vi "CreatePaths_OpenFiles.vi"(8 "error in (no error)":errorcluster, 11 "HDF5_file_refs in":T2={"base path"=path "", "PathNow1"=path "", "PathNow2"=path "", "DateNow"="", "NAS path"=path "", "LogFiltStage"=FALSE, "LogNoise_df_1"=FALSE, "LogNoise_df_2"=FALSE, "LogNoise_df_3"=FALSE, "LogNoise_df_4"=FALSE, "Config"={"UsrCfg"={"Paths"={"CfgFile"=path "", "LogFolder"=path "", "LogFile"=path "", "NAS path"=path "", "ThreshFile"=path "", "RedunFolder"=path ""}, "SampleRate"=0.0}, "FP_User"={"#NoiseSums"=0, "Max_df"=1, "AvgAvg"=FALSE, "#Avg"=0, "AutoCenter"=FALSE, "Inclin"={"Vmin"=0.0, "Vmax"=0.0, "Angle_min"=0.0, "Angle_max"=0.0, "Offset"=0.0, "Pos_Neg"=FALSE}, "1"={"Cal_"={"Fine"=0.0, "Coarse_"=0.0}, "Beac"={"Fine"=0.0, "Coarse_"=0.0}, "Scale"={"Step4"=0.0, "Step5"=0.0, "Step6"=0.0, "Step7"=0.0}, "Offset"=0.0, "Scale_Noise"=0.0, "Scale_Step1"=0.0, "Scale_In_RT"=0.0, "ScaleMeas"=0.0, "FreqsToRemove"=[], "Width"=[0, 1633], "ScaleMeasEnum"=enum."1", "FilterEnab"=enum."Step 1"}, "2"={"Cal_"={"Fine"=0.0, "Coarse_"=0.0}, "Beac"={"Fine"=0.0, "Coarse_"=0.0}, "Scale"={"Step4"=0.0, "Step5"=0.0, "Step6"=0.0, "Step7"=0.0}, "Offset"=0.0, "Scale_Noise"=0.0, "Scale_Step1"=0.0, "Scale_In_RT"=0.0, "ScaleMeas"=0.0, "FreqsToRemove"=[], "Width"=[0, 1633], "ScaleMeasEnum"=enum."1", "FilterEnab"=enum."Step 1"}, "3"={"Cal_"={"Fine"=0.0, "Coarse_"=0.0}, "Beac"={"Fine"=0.0, "Coarse_"=0.0}, "Scale"={"Step4"=0.0, "Step5"=0.0, "Step6"=0.0, "Step7"=0.0}, "Offset"=0.0, "Scale_Noise"=0.0, "Scale_Step1"=0.0, "Scale_In_RT"=0.0, "ScaleMeas"=0.0, "FreqsToRemove"=[], "Width"=[0, 1633], "ScaleMeasEnum"=enum."1", "FilterEnab"=enum."Step 1"}, "4"={"Cal_"={"Fine"=0.0, "Coarse_"=0.0}, "Beac"={"Fine"=0.0, "Coarse_"=0.0}, "Scale"={"Step4"=0.0, "Step5"=0.0, "Step6"=0.0, "Step7"=0.0}, "Offset"=0.0, "Scale_Noise"=0.0, "Scale_Step1"=0.0, "Scale_In_RT"=0.0, "ScaleMeas"=0.0, "FreqsToRemove"=[], "Width"=[0, 1633], "ScaleMeasEnum"=enum."1", "FilterEnab"=enum."Step 1"}, "Target to Probe"=enum."1", "SNR_Thresh"=0.0, "Paths"={"CfgFile"=path "", "LogFolder"=path "", "LogFile"=path "", "NAS path"=path "", "ThreshFile"=path "", "RedunFolder"=path ""}, "Connex_Location"="", "SimulateFPGA"=FALSE, "Deadband"=0.0}}, "HDFRefs1"={"File"=0, "ToneRefs"=[], "NoiseRefs"=[], "TC_Refs"={"Group_ref"=0, "TimeString_dset"=0, "TimeStamp_dset"=0, "TC0_LP1_Hi"=0, "TC1_LP1_MidHi"=0, "TC2_LP1_Mid"=0, "TC3_LP1_LoMid"=0, "TC4_LP1_Lo"=0, "TC5_LP2_Hi"=0, "TC6_LP2_MidHi"=0, "TC7_LP2_Mid"=0, "TC8_LP2_LoMid"=0, "TC9_LP2_Lo"=0, "TC10_HVAC_Cond_In"=0, "TC11_HVAC_Cond_Out"=0, "TC12_Gen_Exhaust"=0, "TC13_Tamb_Inter"=0}, "ValidRefs"={"Group_ref"=0, "Weath_Valid_dset"=0, "Disdr_Valid_dset"=0, "Saturat_dset"=0, "Alarm_Valid_dset"=0, "Time_Valid_dset"=0, "Time_AlarmChange_dset"=0, "Alarm_Source_dset"=0}, "DisdromRefs"={"BasicGroup_ref"=0, "TimeStamp_dset"=0, "TotalRainRate_dset"=0, "Liquid_dset"=0, "Solid_dset"=0, "TotalRain_dset"=0, "Visibility_dset"=0, "RadarReflect_dset"=0, "MaxDiam_dset"=0, "MeasdParticles_dset"=0, "ParticlMinSpeed_dset"=0, "ParticlMaxSpeed_dset"=0, "ParticlMinDiam_dset"=0, "NonHydrParticls_dset"=0, "NonHydrVolum_dset"=0, "UnknownParticls_dset"=0, "UnknownVolum_dset"=0, "HydromType_dset"=0, "SpectGroup_ref"=0, "Spectrum_dset"=0, "Status_dset_deprecated"=0}, "TE_Refs"={"Group_ref"=0, "TE_Temp1_dset"=0, "TE_Outp1_dset"=0, "TE_Temp2_dset"=0, "TE_Outp2_dset"=0, "TE_Temp3_dset"=0, "TE_Outp3_dset"=0, "TimeStamp"=0}, "UPS_Refs_Deprecated"={"Group_ref"=0, "TimeString_dset"=0, "TimeStamp_dset"=0, "V_dset"=0, "A_dset"=0, "Hz_dset"=0, "W_dset"=0, "%_dset"=0}, "Weath_Refs"={"Group_ref"=0, "TimeString_dset"=0, "TimeStamp_dset "=0, "WindSpd_dset"=0, "WindGusts_dset"=0, "WindDir_dset"=0, "WindDirSTD_dset"=0, "Temp_dset"=0, "Humidity_dset"=0, "Pressure_dset"=0, "RainRate_dset"=0, "RainFall_dset"=0}, "AI_Refs"={"Group_ref"=0, "TimeString_dset"=0, "TimeStamp_dset"=0, "AI0_dset"=0, "AI1_dset"=0, "AI2_dset"=0, "AI3_dset"=0, "AI4_dset"=0, "AI5_dset"=0, "AI6_dset"=0, "AI16_dset"=0, "AI17_dset"=0, "AI18_dset"=0, "AzStdDev_dset"=0, "AI19_dset"=0, "ElStdDev_dset"=0, "BlowerPwr_dset"=0}, "Filter_Refs"={"Filter_Group_ref"=0, "TimeStamp_dset"=0, "Filter_dset"=0}, "ADAM_Refs"={"Group_ref"=0, "ADAM_CoPol_dset"=0, "ADAM_XPol_dset"=0, "ADAM_Noise_dset"=0, "ADAM_CalBox_dset"=0, "TimeStamp"=0}, "Complex"=[]}, "HDFRefs2"={"File"=0, "ToneRefs"=[], "NoiseRefs"=[], "TC_Refs"={"Group_ref"=0, "TimeString_dset"=0, "TimeStamp_dset"=0, "TC0_LP1_Hi"=0, "TC1_LP1_MidHi"=0, "TC2_LP1_Mid"=0, "TC3_LP1_LoMid"=0, "TC4_LP1_Lo"=0, "TC5_LP2_Hi"=0, "TC6_LP2_MidHi"=0, "TC7_LP2_Mid"=0, "TC8_LP2_LoMid"=0, "TC9_LP2_Lo"=0, "TC10_HVAC_Cond_In"=0, "TC11_HVAC_Cond_Out"=0, "TC12_Gen_Exhaust"=0, "TC13_Tamb_Inter"=0}, "ValidRefs"={"Group_ref"=0, "Weath_Valid_dset"=0, "Disdr_Valid_dset"=0, "Saturat_dset"=0, "Alarm_Valid_dset"=0, "Time_Valid_dset"=0, "Time_AlarmChange_dset"=0, "Alarm_Source_dset"=0}, "DisdromRefs"={"BasicGroup_ref"=0, "TimeStamp_dset"=0, "TotalRainRate_dset"=0, "Liquid_dset"=0, "Solid_dset"=0, "TotalRain_dset"=0, "Visibility_dset"=0, "RadarReflect_dset"=0, "MaxDiam_dset"=0, "MeasdParticles_dset"=0, "ParticlMinSpeed_dset"=0, "ParticlMaxSpeed_dset"=0, "ParticlMinDiam_dset"=0, "NonHydrParticls_dset"=0, "NonHydrVolum_dset"=0, "UnknownParticls_dset"=0, "UnknownVolum_dset"=0, "HydromType_dset"=0, "SpectGroup_ref"=0, "Spectrum_dset"=0, "Status_dset_deprecated"=0}, "TE_Refs"={"Group_ref"=0, "TE_Temp1_dset"=0, "TE_Outp1_dset"=0, "TE_Temp2_dset"=0, "TE_Outp2_dset"=0, "TE_Temp3_dset"=0, "TE_Outp3_dset"=0, "TimeStamp"=0}, "UPS_Refs_Deprecated"={"Group_ref"=0, "TimeString_dset"=0, "TimeStamp_dset"=0, "V_dset"=0, "A_dset"=0, "Hz_dset"=0, "W_dset"=0, "%_dset"=0}, "Weath_Refs"={"Group_ref"=0, "TimeString_dset"=0, "TimeStamp_dset "=0, "WindSpd_dset"=0, "WindGusts_dset"=0, "WindDir_dset"=0, "WindDirSTD_dset"=0, "Temp_dset"=0, "Humidity_dset"=0, "Pressure_dset"=0, "RainRate_dset"=0, "RainFall_dset"=0}, "AI_Refs"={"Group_ref"=0, "TimeString_dset"=0, "TimeStamp_dset"=0, "AI0_dset"=0, "AI1_dset"=0, "AI2_dset"=0, "AI3_dset"=0, "AI4_dset"=0, "AI5_dset"=0, "AI6_dset"=0, "AI16_dset"=0, "AI17_dset"=0, "AI18_dset"=0, "AzStdDev_dset"=0, "AI19_dset"=0, "ElStdDev_dset"=0, "BlowerPwr_dset"=0}, "Filter_Refs"={"Filter_Group_ref"=0, "TimeStamp_dset"=0, "Filter_dset"=0}, "ADAM_Refs"={"Group_ref"=0, "ADAM_CoPol_dset"=0, "ADAM_XPol_dset"=0, "ADAM_Noise_dset"=0, "ADAM_CalBox_dset"=0, "TimeStamp"=0}, "Complex"=[]}, "LogData"={"Tone"=[], "TCData"={"TimeStamp"=0.0, "TimeString"="", "TC0_LP1_Hi"=0.0, "TC1_LP1_MidHi"=0.0, "TC2_LP1_Mid"=0.0, "TC3_LP1_LoMid"=0.0, "TC4_LP1_Lo"=0.0, "TC5_LP2_Hi"=0.0, "TC6_LP2_MidHi"=0.0, "TC7_LP2_Mid"=0.0, "TC8_LP2_LoMid"=0.0, "TC9_LP2_Lo"=0.0, "TC10_HVAC_Cond_In"=0.0, "TC11_HVAC_Cond_Out"=0.0, "TC12_Gen_Exhaust"=0.0, "TC13_Amb_Inter"=0.0, "TC14_Unused"=0.0, "TC15_Unused"=0.0, "TC16_Unused"=0.0, "TC17_Unused"=0.0, "TC18_Unused"=0.0, "TC19_Unused"=0.0, "TC20_Unused"=0.0, "TC21_Unused"=0.0, "TC22_Unused"=0.0, "TC23_Unused"=0.0, "TC24_Unused"=0.0, "TC25_Unused"=0.0, "TC26_Unused"=0.0, "TC27_Unused"=0.0, "TC28_Unused"=0.0, "TC29_Unused"=0.0, "TC30_Unused"=0.0, "TC31_Unused"=0.0}, "AI"={"TimeString"="", "Time Stamp"=0.0, "AI0_Unused"=0.0, "AI1_-5V"=0.0, "AI2_+5V"=0.0, "AI3_+6V"=0.0, "AI4_+12V"=0.0, "AI5_+15V"=0.0, "AI6_+28V"=0.0, "AI7_Unused"=0.0, "Ai16_72GHz_CalPower"=0.0, "Ai17_84GHz_CalPower"=0.0, "Ai18_InclinAz"=0.0, "Ai19_InclinEl"=0.0, "Ai20_BlowerPwr"=0.0, "Ai21_Unused"=0.0, "Ai22_Unused"=0.0, "Ai23_Unused"=0.0, "InclinA_StdDev"=0.0, "InclinB_StdDev"=0.0, "InclinAz_Unfilt"=0.0, "InclinEl_Unfilt"=0.0}, "NoiseTrace"=[], "NoiseInfo"=[], "Disdrom"=[], "Weath"=[], "TE"={"TimeString"="", "TimeStamp"=0.0, "Temp"=0.0, "Output"=0.0, "Temp 2"=0.0, "Output 2"=0.0, "Temp 3"=0.0, "Output 3"=0.0}, "ADAM"={"Timestamp"=0.0, "Time string"="", "Fault 1"=FALSE, "Fault 2"=FALSE, "Fault 3"=FALSE, "Fault 4"=FALSE, "Fault 5"=FALSE, "Fault 6"=FALSE, "Value 1"=0.0, "Value 2"=0.0, "Value 3"=0.0, "Value 4"=0.0, "Value 5"=0.0, "Value 6"=0.0}, "TimeDomain"=[]}, "AlarmCfg"={"TC13"={"Enbl"=FALSE, "ErrsAndWarns"={0.0, 5.663716814159292, 7.168141592920354, 8.584070796460177}}, "AI1"={"Enbl"=FALSE, "ErrsAndWarns"={0.0, 5.663716814159292, 7.168141592920354, 8.584070796460177}}, "AI2"={"Enbl"=FALSE, "ErrsAndWarns"={0.0, 5.663716814159292, 7.168141592920354, 8.584070796460177}}, "AI3"={"Enbl"=FALSE, "ErrsAndWarns"={0.0, 5.663716814159292, 7.168141592920354, 8.584070796460177}}, "AI4"={"Enbl"=FALSE, "ErrsAndWarns"={0.0, 5.663716814159292, 7.168141592920354, 8.584070796460177}}, "AI5"={"Enbl"=FALSE, "ErrsAndWarns"={0.0, 5.663716814159292, 7.168141592920354, 8.584070796460177}}, "AI6"={"Enbl"=FALSE, "ErrsAndWarns"={0.0, 5.663716814159292, 7.168141592920354, 8.584070796460177}}, "AI18"={"Enbl"=FALSE, "ErrsAndWarns"={0.0, 5.663716814159292, 7.168141592920354, 8.584070796460177}}, "AI19"={"Enbl"=FALSE, "ErrsAndWarns"={0.0, 5.663716814159292, 7.168141592920354, 8.584070796460177}}, "TE1"={"Enbl"=FALSE, "ErrsAndWarns"={0.0, 5.663716814159292, 7.168141592920354, 8.584070796460177}}, "TE2"={"Enbl"=TRUE, "ErrsAndWarns"={0.0, 5.663716814159292, 7.168141592920354, 8.584070796460177}}, "TE3"={"Enbl"=FALSE, "ErrsAndWarns"={0.0, 5.663716814159292, 7.168141592920354, 8.584070796460177}}, "ADAM1"={"Enbl"=FALSE, "ErrsAndWarns"={0.0, 5.663716814159292, 7.168141592920354, 8.584070796460177}}, "ADAM2"={"Enbl"=FALSE, "ErrsAndWarns"={0.0, 5.663716814159292, 7.168141592920354, 8.584070796460177}}, "ADAM3"={"Enbl"=FALSE, "ErrsAndWarns"={0.0, 5.663716814159292, 7.168141592920354, 8.584070796460177}}, "ADAM4"={"Enbl"=FALSE, "ErrsAndWarns"={0.0, 5.663716814159292, 7.168141592920354, 8.584070796460177}}, "72CoBeacFreq"={"Enbl"=FALSE, "ErrsAndWarns"={0.0, 5.663716814159292, 7.168141592920354, 8.584070796460177}}, "72CoCalFreq"={"Enbl"=FALSE, "ErrsAndWarns"={0.0, 5.663716814159292, 7.168141592920354, 8.584070796460177}}, "84CoBeacFreq"={"Enbl"=FALSE, "ErrsAndWarns"={0.0, 5.663716814159292, 7.168141592920354, 8.584070796460177}}, "84CoCalFreq"={"Enbl"=FALSE, "ErrsAndWarns"={0.0, 5.663716814159292, 7.168141592920354, 8.584070796460177}}, "72Co_CalTonePwr"={"Enbl"=FALSE, "ErrsAndWarns"={0.0, 5.663716814159292, 7.168141592920354, 8.584070796460177}}, "72X_CalTonePwr"={"Enbl"=FALSE, "ErrsAndWarns"={0.0, 5.663716814159292, 7.168141592920354, 8.584070796460177}}, "84Co_CalTonePwr"={"Enbl"=FALSE, "ErrsAndWarns"={0.0, 5.663716814159292, 7.168141592920354, 8.584070796460177}}, "84X_CalTonePwr"={"Enbl"=FALSE, "ErrsAndWarns"={0.0, 5.663716814159292, 7.168141592920354, 8.584070796460177}}}, "DO"=[], "AllAlarms"=[], "Alarm Status"={"Green"=FALSE, "Rx_Yell"=FALSE, "Cx_Yell"=FALSE, "Red"=FALSE, "Source"=""}, "SaturationStatus"={"84"=[], "72"=[]}, "WeatherStatus"=[], "10HzRefs"={"72Co_dset"=0, "84Co_dset"=0, "FileRef"=0}} {"10HzRefs"."FileRef" format="%.0x"; "10HzRefs"."84Co_dset" format="%.0x"; "10HzRefs"."72Co_dset" format="%.0x"; "AlarmCfg"."84X_CalTonePwr"."ErrsAndWarns" scale=-120.0..-45.0; "AlarmCfg"."72X_CalTonePwr"."ErrsAndWarns" scale=-120.0..-45.0; "AlarmCfg"."84Co_CalTonePwr"."ErrsAndWarns" scale=-120.0..-45.0; "AlarmCfg"."72Co_CalTonePwr"."ErrsAndWarns" scale=-120.0..-45.0; "AlarmCfg"."84CoCalFreq"."ErrsAndWarns" scale=24.9..25.1; "AlarmCfg"."84CoBeacFreq"."ErrsAndWarns" scale=25.5..27.0; "AlarmCfg"."72CoCalFreq"."ErrsAndWarns" scale=24.9..25.1; "AlarmCfg"."72CoBeacFreq"."ErrsAndWarns" scale=25.5..27.0; "AlarmCfg"."ADAM4"."ErrsAndWarns" scale=30.0..52.0; "AlarmCfg"."ADAM3"."ErrsAndWarns" scale=30.0..52.0; "AlarmCfg"."ADAM2"."ErrsAndWarns" scale=30.0..52.0; "AlarmCfg"."ADAM1"."ErrsAndWarns" scale=30.0..52.0; "AlarmCfg"."TE3"."ErrsAndWarns" scale=30.0..52.0; "AlarmCfg"."TE2"."ErrsAndWarns" scale=30.0..52.0; "AlarmCfg"."TE1"."ErrsAndWarns" scale=20.0..52.0; "AlarmCfg"."AI19"."ErrsAndWarns" scale=0.0..60.0; "AlarmCfg"."AI18"."ErrsAndWarns" scale=-10.0..10.0; "AlarmCfg"."AI6"."ErrsAndWarns" scale=0.0..35.0; "AlarmCfg"."AI5"."ErrsAndWarns" scale=0.0..20.0; "AlarmCfg"."AI4"."ErrsAndWarns" scale=0.0..15.0; "AlarmCfg"."AI3"."ErrsAndWarns" scale=0.0..10.0; "AlarmCfg"."AI2"."ErrsAndWarns" scale=0.0..10.0; "AlarmCfg"."TC13"."ErrsAndWarns" scale=-10.0..40.0; "LogData"."NoiseInfo"."HDF5_NoiseInfo"."Sum" format="%^#.1g"; "HDFRefs2"."Complex"."Group_ref" format="%.0x"; "HDFRefs2"."Complex"."QSpect_dset" format="%.0x"; "HDFRefs2"."Complex"."ISpect_dset" format="%.0x"; "HDFRefs2"."Complex"."PwrSpect_dset" format="%.0x"; "HDFRefs2"."Complex"."TImeStamp_dset" format="%.0x"; "HDFRefs2"."ADAM_Refs"."Group_ref" format="%.0x"; "HDFRefs2"."ADAM_Refs"."ADAM_CoPol_dset" format="%.0x"; "HDFRefs2"."ADAM_Refs"."ADAM_XPol_dset" format="%.0x"; "HDFRefs2"."ADAM_Refs"."ADAM_Noise_dset" format="%.0x"; "HDFRefs2"."ADAM_Refs"."ADAM_CalBox_dset" format="%.0x"; "HDFRefs2"."ADAM_Refs"."TimeStamp" format="%.0x"; "HDFRefs2"."Filter_Refs"."Filter_Group_ref" format="%.0x"; "HDFRefs2"."Filter_Refs"."TimeStamp_dset" format="%.0x"; "HDFRefs2"."Filter_Refs"."Filter_dset" format="%.0x"; "HDFRefs2"."AI_Refs"."BlowerPwr_dset" format="%.0x"; "HDFRefs2"."AI_Refs"."ElStdDev_dset" format="%.0x"; "HDFRefs2"."AI_Refs"."AzStdDev_dset" format="%.0x"; "HDFRefs2"."AI_Refs"."AI19_dset" format="%.0x"; "HDFRefs2"."AI_Refs"."AI18_dset" format="%.0x"; "HDFRefs2"."AI_Refs"."AI17_dset" format="%.0x"; "HDFRefs2"."AI_Refs"."AI16_dset" format="%.0x"; "HDFRefs2"."AI_Refs"."AI6_dset" format="%.0x"; "HDFRefs2"."AI_Refs"."AI5_dset" format="%.0x"; "HDFRefs2"."AI_Refs"."AI4_dset" format="%.0x"; "HDFRefs2"."AI_Refs"."AI3_dset" format="%.0x"; "HDFRefs2"."AI_Refs"."AI2_dset" format="%.0x"; "HDFRefs2"."AI_Refs"."AI0_dset" format="%.0x"; "HDFRefs2"."AI_Refs"."AI1_dset" format="%.0x"; "HDFRefs2"."AI_Refs"."TimeString_dset" format="%.0x"; "HDFRefs2"."AI_Refs"."TimeStamp_dset" format="%.0x"; "HDFRefs2"."AI_Refs"."Group_ref" format="%.0x"; "HDFRefs2"."Weath_Refs"."WindDirSTD_dset" format="%.0x"; "HDFRefs2"."Weath_Refs"."WindGusts_dset" format="%.0x"; "HDFRefs2"."Weath_Refs"."RainFall_dset" format="%.0x"; "HDFRefs2"."Weath_Refs"."RainRate_dset" format="%.0x"; "HDFRefs2"."Weath_Refs"."Pressure_dset" format="%.0x"; "HDFRefs2"."Weath_Refs"."Humidity_dset" format="%.0x"; "HDFRefs2"."Weath_Refs"."Temp_dset" format="%.0x"; "HDFRefs2"."Weath_Refs"."WindDir_dset" format="%.0x"; "HDFRefs2"."Weath_Refs"."WindSpd_dset" format="%.0x"; "HDFRefs2"."Weath_Refs"."TimeStamp_dset" format="%.0x"; "HDFRefs2"."Weath_Refs"."Group_ref" format="%.0x"; "HDFRefs2"."Weath_Refs"."TimeString_dset" format="%.0x"; "HDFRefs2"."UPS_Refs_Deprecated"."TimeStamp_dset" format="%.0x"; "HDFRefs2"."UPS_Refs_Deprecated"."TimeString_dset" format="%.0x"; "HDFRefs2"."UPS_Refs_Deprecated"."%_dset" format="%.0x"; "HDFRefs2"."UPS_Refs_Deprecated"."W_dset" format="%.0x"; "HDFRefs2"."UPS_Refs_Deprecated"."Hz_dset" format="%.0x"; "HDFRefs2"."UPS_Refs_Deprecated"."A_dset" format="%.0x"; "HDFRefs2"."UPS_Refs_Deprecated"."V_dset" format="%.0x"; "HDFRefs2"."UPS_Refs_Deprecated"."Group_ref" format="%.0x"; "HDFRefs2"."TE_Refs"."TimeStamp" format="%.0x"; "HDFRefs2"."TE_Refs"."TE_Outp3_dset" format="%.0x"; "HDFRefs2"."TE_Refs"."TE_Temp3_dset" format="%.0x"; "HDFRefs2"."TE_Refs"."TE_Outp2_dset" format="%.0x"; "HDFRefs2"."TE_Refs"."TE_Temp2_dset" format="%.0x"; "HDFRefs2"."TE_Refs"."TE_Outp1_dset" format="%.0x"; "HDFRefs2"."TE_Refs"."TE_Temp1_dset" format="%.0x"; "HDFRefs2"."TE_Refs"."Group_ref" format="%.0x"; "HDFRefs2"."DisdromRefs"."Status_dset_deprecated" format="%.0x"; "HDFRefs2"."DisdromRefs"."Spectrum_dset" format="%.0x"; "HDFRefs2"."DisdromRefs"."SpectGroup_ref" format="%.0x"; "HDFRefs2"."DisdromRefs"."HydromType_dset" format="%.0x"; "HDFRefs2"."DisdromRefs"."UnknownVolum_dset" format="%.0x"; "HDFRefs2"."DisdromRefs"."UnknownParticls_dset" format="%.0x"; "HDFRefs2"."DisdromRefs"."NonHydrVolum_dset" format="%.0x"; "HDFRefs2"."DisdromRefs"."NonHydrParticls_dset" format="%.0x"; "HDFRefs2"."DisdromRefs"."ParticlMinDiam_dset" format="%.0x"; "HDFRefs2"."DisdromRefs"."ParticlMaxSpeed_dset" format="%.0x"; "HDFRefs2"."DisdromRefs"."RadarReflect_dset" format="%.0x"; "HDFRefs2"."DisdromRefs"."Visibility_dset" format="%.0x"; "HDFRefs2"."DisdromRefs"."TotalRain_dset" format="%.0x"; "HDFRefs2"."DisdromRefs"."Solid_dset" format="%.0x"; "HDFRefs2"."DisdromRefs"."Liquid_dset" format="%.0x"; "HDFRefs2"."DisdromRefs"."TotalRainRate_dset" format="%.0x"; "HDFRefs2"."DisdromRefs"."TimeStamp_dset" format="%.0x"; "HDFRefs2"."DisdromRefs"."ParticlMinSpeed_dset" format="%.0x"; "HDFRefs2"."DisdromRefs"."MeasdParticles_dset" format="%.0x"; "HDFRefs2"."DisdromRefs"."MaxDiam_dset" format="%.0x"; "HDFRefs2"."DisdromRefs"."BasicGroup_ref" format="%.0x"; "HDFRefs2"."ValidRefs"."Alarm_Source_dset" format="%.0x"; "HDFRefs2"."ValidRefs"."Time_AlarmChange_dset" format="%.0x"; "HDFRefs2"."ValidRefs"."Time_Valid_dset" format="%.0x"; "HDFRefs2"."ValidRefs"."Alarm_Valid_dset" format="%.0x"; "HDFRefs2"."ValidRefs"."Saturat_dset" format="%.0x"; "HDFRefs2"."ValidRefs"."Group_ref" format="%.0x"; "HDFRefs2"."ValidRefs"."Weath_Valid_dset" format="%.0x"; "HDFRefs2"."ValidRefs"."Disdr_Valid_dset" format="%.0x"; "HDFRefs2"."TC_Refs"."TC13_Tamb_Inter" format="%.0x"; "HDFRefs2"."TC_Refs"."TC12_Gen_Exhaust" format="%.0x"; "HDFRefs2"."TC_Refs"."TC11_HVAC_Cond_Out" format="%.0x"; "HDFRefs2"."TC_Refs"."TC10_HVAC_Cond_In" format="%.0x"; "HDFRefs2"."TC_Refs"."TC9_LP2_Lo" format="%.0x"; "HDFRefs2"."TC_Refs"."TC8_LP2_LoMid" format="%.0x"; "HDFRefs2"."TC_Refs"."TC7_LP2_Mid" format="%.0x"; "HDFRefs2"."TC_Refs"."TC6_LP2_MidHi" format="%.0x"; "HDFRefs2"."TC_Refs"."TC5_LP2_Hi" format="%.0x"; "HDFRefs2"."TC_Refs"."TC4_LP1_Lo" format="%.0x"; "HDFRefs2"."TC_Refs"."TC3_LP1_LoMid" format="%.0x"; "HDFRefs2"."TC_Refs"."TC2_LP1_Mid" format="%.0x"; "HDFRefs2"."TC_Refs"."TC1_LP1_MidHi" format="%.0x"; "HDFRefs2"."TC_Refs"."TC0_LP1_Hi" format="%.0x"; "HDFRefs2"."TC_Refs"."TimeString_dset" format="%.0x"; "HDFRefs2"."TC_Refs"."TimeStamp_dset" format="%.0x"; "HDFRefs2"."TC_Refs"."Group_ref" format="%.0x"; "HDFRefs2"."NoiseRefs"."TimeStamp_df_dset" format="%.0x"; "HDFRefs2"."NoiseRefs"."sum_dset" format="%.0x"; "HDFRefs2"."NoiseRefs"."df_dset" format="%.0x"; "HDFRefs2"."NoiseRefs"."TimeStamp_dset" format="%.0x"; "HDFRefs2"."NoiseRefs"."SumdSpectrum_dset" format="%.0x"; "HDFRefs2"."NoiseRefs"."TimeString_dset" format="%.0x"; "HDFRefs2"."NoiseRefs"."Group_ref" format="%.0x"; "HDFRefs2"."ToneRefs"."Group_ref" format="%.0x"; "HDFRefs2"."ToneRefs"."Cal"."Downshift_dset" format="%.0x"; "HDFRefs2"."ToneRefs"."Cal"."DeltaPhase_dset" format="%.0x"; "HDFRefs2"."ToneRefs"."Cal"."Phase_dset" format="%.0x"; "HDFRefs2"."ToneRefs"."Cal"."SNR_dset" format="%.0x"; "HDFRefs2"."ToneRefs"."Cal"."df_dset" format="%.0x"; "HDFRefs2"."ToneRefs"."Cal"."PeakLoc_dset" format="%.0x"; "HDFRefs2"."ToneRefs"."Cal"."MaxValue_dset" format="%.0x"; "HDFRefs2"."ToneRefs"."Cal"."TImeStamp_dset" format="%.0x"; "HDFRefs2"."ToneRefs"."Cal"."TimeString_dset" format="%.0x"; "HDFRefs2"."ToneRefs"."Beac"."Downshift_dset" format="%.0x"; "HDFRefs2"."ToneRefs"."Beac"."DeltaPhase_dset" format="%.0x"; "HDFRefs2"."ToneRefs"."Beac"."Phase_dset" format="%.0x"; "HDFRefs2"."ToneRefs"."Beac"."SNR_dset" format="%.0x"; "HDFRefs2"."ToneRefs"."Beac"."df_dset" format="%.0x"; "HDFRefs2"."ToneRefs"."Beac"."PeakLoc_dset" format="%.0x"; "HDFRefs2"."ToneRefs"."Beac"."MaxValue_dset" format="%.0x"; "HDFRefs2"."ToneRefs"."Beac"."TImeStamp_dset" format="%.0x"; "HDFRefs2"."ToneRefs"."Beac"."TimeString_dset" format="%.0x"; "HDFRefs2"."ToneRefs"."CalZoom_dSet" format="%.0x"; "HDFRefs2"."ToneRefs"."BeacZoom_dSet" format="%.0x"; "HDFRefs2"."File" format="%.0x"; "HDFRefs1"."Complex"."Group_ref" format="%.0x"; "HDFRefs1"."Complex"."QSpect_dset" format="%.0x"; "HDFRefs1"."Complex"."ISpect_dset" format="%.0x"; "HDFRefs1"."Complex"."PwrSpect_dset" format="%.0x"; "HDFRefs1"."Complex"."TImeStamp_dset" format="%.0x"; "HDFRefs1"."ADAM_Refs"."Group_ref" format="%.0x"; "HDFRefs1"."ADAM_Refs"."ADAM_CoPol_dset" format="%.0x"; "HDFRefs1"."ADAM_Refs"."ADAM_XPol_dset" format="%.0x"; "HDFRefs1"."ADAM_Refs"."ADAM_Noise_dset" format="%.0x"; "HDFRefs1"."ADAM_Refs"."ADAM_CalBox_dset" format="%.0x"; "HDFRefs1"."ADAM_Refs"."TimeStamp" format="%.0x"; "HDFRefs1"."Filter_Refs"."Filter_Group_ref" format="%.0x"; "HDFRefs1"."Filter_Refs"."TimeStamp_dset" format="%.0x"; "HDFRefs1"."Filter_Refs"."Filter_dset" format="%.0x"; "HDFRefs1"."AI_Refs"."BlowerPwr_dset" format="%.0x"; "HDFRefs1"."AI_Refs"."ElStdDev_dset" format="%.0x"; "HDFRefs1"."AI_Refs"."AzStdDev_dset" format="%.0x"; "HDFRefs1"."AI_Refs"."AI19_dset" format="%.0x"; "HDFRefs1"."AI_Refs"."AI18_dset" format="%.0x"; "HDFRefs1"."AI_Refs"."AI17_dset" format="%.0x"; "HDFRefs1"."AI_Refs"."AI16_dset" format="%.0x"; "HDFRefs1"."AI_Refs"."AI6_dset" format="%.0x"; "HDFRefs1"."AI_Refs"."AI5_dset" format="%.0x"; "HDFRefs1"."AI_Refs"."AI4_dset" format="%.0x"; "HDFRefs1"."AI_Refs"."AI3_dset" format="%.0x"; "HDFRefs1"."AI_Refs"."AI2_dset" format="%.0x"; "HDFRefs1"."AI_Refs"."AI0_dset" format="%.0x"; "HDFRefs1"."AI_Refs"."AI1_dset" format="%.0x"; "HDFRefs1"."AI_Refs"."TimeString_dset" format="%.0x"; "HDFRefs1"."AI_Refs"."TimeStamp_dset" format="%.0x"; "HDFRefs1"."AI_Refs"."Group_ref" format="%.0x"; "HDFRefs1"."Weath_Refs"."WindDirSTD_dset" format="%.0x"; "HDFRefs1"."Weath_Refs"."WindGusts_dset" format="%.0x"; "HDFRefs1"."Weath_Refs"."RainFall_dset" format="%.0x"; "HDFRefs1"."Weath_Refs"."RainRate_dset" format="%.0x"; "HDFRefs1"."Weath_Refs"."Pressure_dset" format="%.0x"; "HDFRefs1"."Weath_Refs"."Humidity_dset" format="%.0x"; "HDFRefs1"."Weath_Refs"."Temp_dset" format="%.0x"; "HDFRefs1"."Weath_Refs"."WindDir_dset" format="%.0x"; "HDFRefs1"."Weath_Refs"."WindSpd_dset" format="%.0x"; "HDFRefs1"."Weath_Refs"."TimeStamp_dset" format="%.0x"; "HDFRefs1"."Weath_Refs"."Group_ref" format="%.0x"; "HDFRefs1"."Weath_Refs"."TimeString_dset" format="%.0x"; "HDFRefs1"."UPS_Refs_Deprecated"."TimeStamp_dset" format="%.0x"; "HDFRefs1"."UPS_Refs_Deprecated"."TimeString_dset" format="%.0x"; "HDFRefs1"."UPS_Refs_Deprecated"."%_dset" format="%.0x"; "HDFRefs1"."UPS_Refs_Deprecated"."W_dset" format="%.0x"; "HDFRefs1"."UPS_Refs_Deprecated"."Hz_dset" format="%.0x"; "HDFRefs1"."UPS_Refs_Deprecated"."A_dset" format="%.0x"; "HDFRefs1"."UPS_Refs_Deprecated"."V_dset" format="%.0x"; "HDFRefs1"."UPS_Refs_Deprecated"."Group_ref" format="%.0x"; "HDFRefs1"."TE_Refs"."TimeStamp" format="%.0x"; "HDFRefs1"."TE_Refs"."TE_Outp3_dset" format="%.0x"; "HDFRefs1"."TE_Refs"."TE_Temp3_dset" format="%.0x"; "HDFRefs1"."TE_Refs"."TE_Outp2_dset" format="%.0x"; "HDFRefs1"."TE_Refs"."TE_Temp2_dset" format="%.0x"; "HDFRefs1"."TE_Refs"."TE_Outp1_dset" format="%.0x"; "HDFRefs1"."TE_Refs"."TE_Temp1_dset" format="%.0x"; "HDFRefs1"."TE_Refs"."Group_ref" format="%.0x"; "HDFRefs1"."DisdromRefs"."Status_dset_deprecated" format="%.0x"; "HDFRefs1"."DisdromRefs"."Spectrum_dset" format="%.0x"; "HDFRefs1"."DisdromRefs"."SpectGroup_ref" format="%.0x"; "HDFRefs1"."DisdromRefs"."HydromType_dset" format="%.0x"; "HDFRefs1"."DisdromRefs"."UnknownVolum_dset" format="%.0x"; "HDFRefs1"."DisdromRefs"."UnknownParticls_dset" format="%.0x"; "HDFRefs1"."DisdromRefs"."NonHydrVolum_dset" format="%.0x"; "HDFRefs1"."DisdromRefs"."NonHydrParticls_dset" format="%.0x"; "HDFRefs1"."DisdromRefs"."ParticlMinDiam_dset" format="%.0x"; "HDFRefs1"."DisdromRefs"."ParticlMaxSpeed_dset" format="%.0x"; "HDFRefs1"."DisdromRefs"."RadarReflect_dset" format="%.0x"; "HDFRefs1"."DisdromRefs"."Visibility_dset" format="%.0x"; "HDFRefs1"."DisdromRefs"."TotalRain_dset" format="%.0x"; "HDFRefs1"."DisdromRefs"."Solid_dset" format="%.0x"; "HDFRefs1"."DisdromRefs"."Liquid_dset" format="%.0x"; "HDFRefs1"."DisdromRefs"."TotalRainRate_dset" format="%.0x"; "HDFRefs1"."DisdromRefs"."TimeStamp_dset" format="%.0x"; "HDFRefs1"."DisdromRefs"."ParticlMinSpeed_dset" format="%.0x"; "HDFRefs1"."DisdromRefs"."MeasdParticles_dset" format="%.0x"; "HDFRefs1"."DisdromRefs"."MaxDiam_dset" format="%.0x"; "HDFRefs1"."DisdromRefs"."BasicGroup_ref" format="%.0x"; "HDFRefs1"."ValidRefs"."Alarm_Source_dset" format="%.0x"; "HDFRefs1"."ValidRefs"."Time_AlarmChange_dset" format="%.0x"; "HDFRefs1"."ValidRefs"."Time_Valid_dset" format="%.0x"; "HDFRefs1"."ValidRefs"."Alarm_Valid_dset" format="%.0x"; "HDFRefs1"."ValidRefs"."Saturat_dset" format="%.0x"; "HDFRefs1"."ValidRefs"."Group_ref" format="%.0x"; "HDFRefs1"."ValidRefs"."Weath_Valid_dset" format="%.0x"; "HDFRefs1"."ValidRefs"."Disdr_Valid_dset" format="%.0x"; "HDFRefs1"."TC_Refs"."TC13_Tamb_Inter" format="%.0x"; "HDFRefs1"."TC_Refs"."TC12_Gen_Exhaust" format="%.0x"; "HDFRefs1"."TC_Refs"."TC11_HVAC_Cond_Out" format="%.0x"; "HDFRefs1"."TC_Refs"."TC10_HVAC_Cond_In" format="%.0x"; "HDFRefs1"."TC_Refs"."TC9_LP2_Lo" format="%.0x"; "HDFRefs1"."TC_Refs"."TC8_LP2_LoMid" format="%.0x"; "HDFRefs1"."TC_Refs"."TC7_LP2_Mid" format="%.0x"; "HDFRefs1"."TC_Refs"."TC6_LP2_MidHi" format="%.0x"; "HDFRefs1"."TC_Refs"."TC5_LP2_Hi" format="%.0x"; "HDFRefs1"."TC_Refs"."TC4_LP1_Lo" format="%.0x"; "HDFRefs1"."TC_Refs"."TC3_LP1_LoMid" format="%.0x"; "HDFRefs1"."TC_Refs"."TC2_LP1_Mid" format="%.0x"; "HDFRefs1"."TC_Refs"."TC1_LP1_MidHi" format="%.0x"; "HDFRefs1"."TC_Refs"."TC0_LP1_Hi" format="%.0x"; "HDFRefs1"."TC_Refs"."TimeString_dset" format="%.0x"; "HDFRefs1"."TC_Refs"."TimeStamp_dset" format="%.0x"; "HDFRefs1"."TC_Refs"."Group_ref" format="%.0x"; "HDFRefs1"."NoiseRefs"."TimeStamp_df_dset" format="%.0x"; "HDFRefs1"."NoiseRefs"."sum_dset" format="%.0x"; "HDFRefs1"."NoiseRefs"."df_dset" format="%.0x"; "HDFRefs1"."NoiseRefs"."TimeStamp_dset" format="%.0x"; "HDFRefs1"."NoiseRefs"."SumdSpectrum_dset" format="%.0x"; "HDFRefs1"."NoiseRefs"."TimeString_dset" format="%.0x"; "HDFRefs1"."NoiseRefs"."Group_ref" format="%.0x"; "HDFRefs1"."ToneRefs"."Group_ref" format="%.0x"; "HDFRefs1"."ToneRefs"."Cal"."Downshift_dset" format="%.0x"; "HDFRefs1"."ToneRefs"."Cal"."DeltaPhase_dset" format="%.0x"; "HDFRefs1"."ToneRefs"."Cal"."Phase_dset" format="%.0x"; "HDFRefs1"."ToneRefs"."Cal"."SNR_dset" format="%.0x"; "HDFRefs1"."ToneRefs"."Cal"."df_dset" format="%.0x"; "HDFRefs1"."ToneRefs"."Cal"."PeakLoc_dset" format="%.0x"; "HDFRefs1"."ToneRefs"."Cal"."MaxValue_dset" format="%.0x"; "HDFRefs1"."ToneRefs"."Cal"."TImeStamp_dset" format="%.0x"; "HDFRefs1"."ToneRefs"."Cal"."TimeString_dset" format="%.0x"; "HDFRefs1"."ToneRefs"."Beac"."Downshift_dset" format="%.0x"; "HDFRefs1"."ToneRefs"."Beac"."DeltaPhase_dset" format="%.0x"; "HDFRefs1"."ToneRefs"."Beac"."Phase_dset" format="%.0x"; "HDFRefs1"."ToneRefs"."Beac"."SNR_dset" format="%.0x"; "HDFRefs1"."ToneRefs"."Beac"."df_dset" format="%.0x"; "HDFRefs1"."ToneRefs"."Beac"."PeakLoc_dset" format="%.0x"; "HDFRefs1"."ToneRefs"."Beac"."MaxValue_dset" format="%.0x"; "HDFRefs1"."ToneRefs"."Beac"."TImeStamp_dset" format="%.0x"; "HDFRefs1"."ToneRefs"."Beac"."TimeString_dset" format="%.0x"; "HDFRefs1"."ToneRefs"."CalZoom_dSet" format="%.0x"; "HDFRefs1"."ToneRefs"."BeacZoom_dSet" format="%.0x"; "HDFRefs1"."File" format="%.0x"; "Config"."FP_User"."Deadband" format="%#.0f"}) -> (0 "error out":errorcluster, 1 "redundant file ref":T1 format="%.0x", 2 "file exists? 2":bool, 3 "data file ref":T1 format="%.0x", 4 "file exists?":bool, 5 "HDF5_file_refs out":T2={"base path"=path "", "PathNow1"=path "", "PathNow2"=path "", "DateNow"="", "NAS path"=path "", "LogFiltStage"=FALSE, "LogNoise_df_1"=FALSE, "LogNoise_df_2"=FALSE, "LogNoise_df_3"=FALSE, "LogNoise_df_4"=FALSE, "Config"={"UsrCfg"={"Paths"={"CfgFile"=path "", "LogFolder"=path "", "LogFile"=path "", "NAS path"=path "", "ThreshFile"=path "", "RedunFolder"=path ""}, "SampleRate"=0.0}, "FP_User"={"#NoiseSums"=0, "Max_df"=1, "AvgAvg"=FALSE, "#Avg"=0, "AutoCenter"=FALSE, "Inclin"={"Vmin"=0.0, "Vmax"=0.0, "Angle_min"=0.0, "Angle_max"=0.0, "Offset"=0.0, "Pos_Neg"=FALSE}, "1"={"Cal_"={"Fine"=0.0, "Coarse_"=0.0}, "Beac"={"Fine"=0.0, "Coarse_"=0.0}, "Scale"={"Step4"=0.0, "Step5"=0.0, "Step6"=0.0, "Step7"=0.0}, "Offset"=0.0, "Scale_Noise"=0.0, "Scale_Step1"=0.0, "Scale_In_RT"=0.0, "ScaleMeas"=0.0, "FreqsToRemove"=[], "Width"=[0, 1633], "ScaleMeasEnum"=enum."1", "FilterEnab"=enum."Step 1"}, "2"={"Cal_"={"Fine"=0.0, "Coarse_"=0.0}, "Beac"={"Fine"=0.0, "Coarse_"=0.0}, "Scale"={"Step4"=0.0, "Step5"=0.0, "Step6"=0.0, "Step7"=0.0}, "Offset"=0.0, "Scale_Noise"=0.0, "Scale_Step1"=0.0, "Scale_In_RT"=0.0, "ScaleMeas"=0.0, "FreqsToRemove"=[], "Width"=[0, 1633], "ScaleMeasEnum"=enum."1", "FilterEnab"=enum."Step 1"}, "3"={"Cal_"={"Fine"=0.0, "Coarse_"=0.0}, "Beac"={"Fine"=0.0, "Coarse_"=0.0}, "Scale"={"Step4"=0.0, "Step5"=0.0, "Step6"=0.0, "Step7"=0.0}, "Offset"=0.0, "Scale_Noise"=0.0, "Scale_Step1"=0.0, "Scale_In_RT"=0.0, "ScaleMeas"=0.0, "FreqsToRemove"=[], "Width"=[0, 1633], "ScaleMeasEnum"=enum."1", "FilterEnab"=enum."Step 1"}, "4"={"Cal_"={"Fine"=0.0, "Coarse_"=0.0}, "Beac"={"Fine"=0.0, "Coarse_"=0.0}, "Scale"={"Step4"=0.0, "Step5"=0.0, "Step6"=0.0, "Step7"=0.0}, "Offset"=0.0, "Scale_Noise"=0.0, "Scale_Step1"=0.0, "Scale_In_RT"=0.0, "ScaleMeas"=0.0, "FreqsToRemove"=[], "Width"=[0, 1633], "ScaleMeasEnum"=enum."1", "FilterEnab"=enum."Step 1"}, "Target to Probe"=enum."1", "SNR_Thresh"=0.0, "Paths"={"CfgFile"=path "", "LogFolder"=path "", "LogFile"=path "", "NAS path"=path "", "ThreshFile"=path "", "RedunFolder"=path ""}, "Connex_Location"="", "SimulateFPGA"=FALSE, "Deadband"=0.0}}, "HDFRefs1"={"File"=0, "ToneRefs"=[], "NoiseRefs"=[], "TC_Refs"={"Group_ref"=0, "TimeString_dset"=0, "TimeStamp_dset"=0, "TC0_LP1_Hi"=0, "TC1_LP1_MidHi"=0, "TC2_LP1_Mid"=0, "TC3_LP1_LoMid"=0, "TC4_LP1_Lo"=0, "TC5_LP2_Hi"=0, "TC6_LP2_MidHi"=0, "TC7_LP2_Mid"=0, "TC8_LP2_LoMid"=0, "TC9_LP2_Lo"=0, "TC10_HVAC_Cond_In"=0, "TC11_HVAC_Cond_Out"=0, "TC12_Gen_Exhaust"=0, "TC13_Tamb_Inter"=0}, "ValidRefs"={"Group_ref"=0, "Weath_Valid_dset"=0, "Disdr_Valid_dset"=0, "Saturat_dset"=0, "Alarm_Valid_dset"=0, "Time_Valid_dset"=0, "Time_AlarmChange_dset"=0, "Alarm_Source_dset"=0}, "DisdromRefs"={"BasicGroup_ref"=0, "TimeStamp_dset"=0, "TotalRainRate_dset"=0, "Liquid_dset"=0, "Solid_dset"=0, "TotalRain_dset"=0, "Visibility_dset"=0, "RadarReflect_dset"=0, "MaxDiam_dset"=0, "MeasdParticles_dset"=0, "ParticlMinSpeed_dset"=0, "ParticlMaxSpeed_dset"=0, "ParticlMinDiam_dset"=0, "NonHydrParticls_dset"=0, "NonHydrVolum_dset"=0, "UnknownParticls_dset"=0, "UnknownVolum_dset"=0, "HydromType_dset"=0, "SpectGroup_ref"=0, "Spectrum_dset"=0, "Status_dset_deprecated"=0}, "TE_Refs"={"Group_ref"=0, "TE_Temp1_dset"=0, "TE_Outp1_dset"=0, "TE_Temp2_dset"=0, "TE_Outp2_dset"=0, "TE_Temp3_dset"=0, "TE_Outp3_dset"=0, "TimeStamp"=0}, "UPS_Refs_Deprecated"={"Group_ref"=0, "TimeString_dset"=0, "TimeStamp_dset"=0, "V_dset"=0, "A_dset"=0, "Hz_dset"=0, "W_dset"=0, "%_dset"=0}, "Weath_Refs"={"Group_ref"=0, "TimeString_dset"=0, "TimeStamp_dset "=0, "WindSpd_dset"=0, "WindGusts_dset"=0, "WindDir_dset"=0, "WindDirSTD_dset"=0, "Temp_dset"=0, "Humidity_dset"=0, "Pressure_dset"=0, "RainRate_dset"=0, "RainFall_dset"=0}, "AI_Refs"={"Group_ref"=0, "TimeString_dset"=0, "TimeStamp_dset"=0, "AI0_dset"=0, "AI1_dset"=0, "AI2_dset"=0, "AI3_dset"=0, "AI4_dset"=0, "AI5_dset"=0, "AI6_dset"=0, "AI16_dset"=0, "AI17_dset"=0, "AI18_dset"=0, "AzStdDev_dset"=0, "AI19_dset"=0, "ElStdDev_dset"=0, "BlowerPwr_dset"=0}, "Filter_Refs"={"Filter_Group_ref"=0, "TimeStamp_dset"=0, "Filter_dset"=0}, "ADAM_Refs"={"Group_ref"=0, "ADAM_CoPol_dset"=0, "ADAM_XPol_dset"=0, "ADAM_Noise_dset"=0, "ADAM_CalBox_dset"=0, "TimeStamp"=0}, "Complex"=[]}, "HDFRefs2"={"File"=0, "ToneRefs"=[], "NoiseRefs"=[], "TC_Refs"={"Group_ref"=0, "TimeString_dset"=0, "TimeStamp_dset"=0, "TC0_LP1_Hi"=0, "TC1_LP1_MidHi"=0, "TC2_LP1_Mid"=0, "TC3_LP1_LoMid"=0, "TC4_LP1_Lo"=0, "TC5_LP2_Hi"=0, "TC6_LP2_MidHi"=0, "TC7_LP2_Mid"=0, "TC8_LP2_LoMid"=0, "TC9_LP2_Lo"=0, "TC10_HVAC_Cond_In"=0, "TC11_HVAC_Cond_Out"=0, "TC12_Gen_Exhaust"=0, "TC13_Tamb_Inter"=0}, "ValidRefs"={"Group_ref"=0, "Weath_Valid_dset"=0, "Disdr_Valid_dset"=0, "Saturat_dset"=0, "Alarm_Valid_dset"=0, "Time_Valid_dset"=0, "Time_AlarmChange_dset"=0, "Alarm_Source_dset"=0}, "DisdromRefs"={"BasicGroup_ref"=0, "TimeStamp_dset"=0, "TotalRainRate_dset"=0, "Liquid_dset"=0, "Solid_dset"=0, "TotalRain_dset"=0, "Visibility_dset"=0, "RadarReflect_dset"=0, "MaxDiam_dset"=0, "MeasdParticles_dset"=0, "ParticlMinSpeed_dset"=0, "ParticlMaxSpeed_dset"=0, "ParticlMinDiam_dset"=0, "NonHydrParticls_dset"=0, "NonHydrVolum_dset"=0, "UnknownParticls_dset"=0, "UnknownVolum_dset"=0, "HydromType_dset"=0, "SpectGroup_ref"=0, "Spectrum_dset"=0, "Status_dset_deprecated"=0}, "TE_Refs"={"Group_ref"=0, "TE_Temp1_dset"=0, "TE_Outp1_dset"=0, "TE_Temp2_dset"=0, "TE_Outp2_dset"=0, "TE_Temp3_dset"=0, "TE_Outp3_dset"=0, "TimeStamp"=0}, "UPS_Refs_Deprecated"={"Group_ref"=0, "TimeString_dset"=0, "TimeStamp_dset"=0, "V_dset"=0, "A_dset"=0, "Hz_dset"=0, "W_dset"=0, "%_dset"=0}, "Weath_Refs"={"Group_ref"=0, "TimeString_dset"=0, "TimeStamp_dset "=0, "WindSpd_dset"=0, "WindGusts_dset"=0, "WindDir_dset"=0, "WindDirSTD_dset"=0, "Temp_dset"=0, "Humidity_dset"=0, "Pressure_dset"=0, "RainRate_dset"=0, "RainFall_dset"=0}, "AI_Refs"={"Group_ref"=0, "TimeString_dset"=0, "TimeStamp_dset"=0, "AI0_dset"=0, "AI1_dset"=0, "AI2_dset"=0, "AI3_dset"=0, "AI4_dset"=0, "AI5_dset"=0, "AI6_dset"=0, "AI16_dset"=0, "AI17_dset"=0, "AI18_dset"=0, "AzStdDev_dset"=0, "AI19_dset"=0, "ElStdDev_dset"=0, "BlowerPwr_dset"=0}, "Filter_Refs"={"Filter_Group_ref"=0, "TimeStamp_dset"=0, "Filter_dset"=0}, "ADAM_Refs"={"Group_ref"=0, "ADAM_CoPol_dset"=0, "ADAM_XPol_dset"=0, "ADAM_Noise_dset"=0, "ADAM_CalBox_dset"=0, "TimeStamp"=0}, "Complex"=[]}, "LogData"={"Tone"=[], "TCData"={"TimeStamp"=0.0, "TimeString"="", "TC0_LP1_Hi"=0.0, "TC1_LP1_MidHi"=0.0, "TC2_LP1_Mid"=0.0, "TC3_LP1_LoMid"=0.0, "TC4_LP1_Lo"=0.0, "TC5_LP2_Hi"=0.0, "TC6_LP2_MidHi"=0.0, "TC7_LP2_Mid"=0.0, "TC8_LP2_LoMid"=0.0, "TC9_LP2_Lo"=0.0, "TC10_HVAC_Cond_In"=0.0, "TC11_HVAC_Cond_Out"=0.0, "TC12_Gen_Exhaust"=0.0, "TC13_Amb_Inter"=0.0, "TC14_Unused"=0.0, "TC15_Unused"=0.0, "TC16_Unused"=0.0, "TC17_Unused"=0.0, "TC18_Unused"=0.0, "TC19_Unused"=0.0, "TC20_Unused"=0.0, "TC21_Unused"=0.0, "TC22_Unused"=0.0, "TC23_Unused"=0.0, "TC24_Unused"=0.0, "TC25_Unused"=0.0, "TC26_Unused"=0.0, "TC27_Unused"=0.0, "TC28_Unused"=0.0, "TC29_Unused"=0.0, "TC30_Unused"=0.0, "TC31_Unused"=0.0}, "AI"={"TimeString"="", "Time Stamp"=0.0, "AI0_Unused"=0.0, "AI1_-5V"=0.0, "AI2_+5V"=0.0, "AI3_+6V"=0.0, "AI4_+12V"=0.0, "AI5_+15V"=0.0, "AI6_+28V"=0.0, "AI7_Unused"=0.0, "Ai16_72GHz_CalPower"=0.0, "Ai17_84GHz_CalPower"=0.0, "Ai18_InclinAz"=0.0, "Ai19_InclinEl"=0.0, "Ai20_BlowerPwr"=0.0, "Ai21_Unused"=0.0, "Ai22_Unused"=0.0, "Ai23_Unused"=0.0, "InclinA_StdDev"=0.0, "InclinB_StdDev"=0.0, "InclinAz_Unfilt"=0.0, "InclinEl_Unfilt"=0.0}, "NoiseTrace"=[], "NoiseInfo"=[], "Disdrom"=[], "Weath"=[], "TE"={"TimeString"="", "TimeStamp"=0.0, "Temp"=0.0, "Output"=0.0, "Temp 2"=0.0, "Output 2"=0.0, "Temp 3"=0.0, "Output 3"=0.0}, "ADAM"={"Timestamp"=0.0, "Time string"="", "Fault 1"=FALSE, "Fault 2"=FALSE, "Fault 3"=FALSE, "Fault 4"=FALSE, "Fault 5"=FALSE, "Fault 6"=FALSE, "Value 1"=0.0, "Value 2"=0.0, "Value 3"=0.0, "Value 4"=0.0, "Value 5"=0.0, "Value 6"=0.0}, "TimeDomain"=[]}, "AlarmCfg"={"TC13"={"Enbl"=FALSE, "ErrsAndWarns"={0.0, 5.663716814159292, 7.168141592920354, 8.584070796460177}}, "AI1"={"Enbl"=FALSE, "ErrsAndWarns"={0.0, 5.663716814159292, 7.168141592920354, 8.584070796460177}}, "AI2"={"Enbl"=FALSE, "ErrsAndWarns"={0.0, 5.663716814159292, 7.168141592920354, 8.584070796460177}}, "AI3"={"Enbl"=FALSE, "ErrsAndWarns"={0.0, 5.663716814159292, 7.168141592920354, 8.584070796460177}}, "AI4"={"Enbl"=FALSE, "ErrsAndWarns"={0.0, 5.663716814159292, 7.168141592920354, 8.584070796460177}}, "AI5"={"Enbl"=FALSE, "ErrsAndWarns"={0.0, 5.663716814159292, 7.168141592920354, 8.584070796460177}}, "AI6"={"Enbl"=FALSE, "ErrsAndWarns"={0.0, 5.663716814159292, 7.168141592920354, 8.584070796460177}}, "AI18"={"Enbl"=FALSE, "ErrsAndWarns"={0.0, 5.663716814159292, 7.168141592920354, 8.584070796460177}}, "AI19"={"Enbl"=FALSE, "ErrsAndWarns"={0.0, 5.663716814159292, 7.168141592920354, 8.584070796460177}}, "TE1"={"Enbl"=FALSE, "ErrsAndWarns"={0.0, 5.663716814159292, 7.168141592920354, 8.584070796460177}}, "TE2"={"Enbl"=TRUE, "ErrsAndWarns"={0.0, 5.663716814159292, 7.168141592920354, 8.584070796460177}}, "TE3"={"Enbl"=FALSE, "ErrsAndWarns"={0.0, 5.663716814159292, 7.168141592920354, 8.584070796460177}}, "ADAM1"={"Enbl"=FALSE, "ErrsAndWarns"={0.0, 5.663716814159292, 7.168141592920354, 8.584070796460177}}, "ADAM2"={"Enbl"=FALSE, "ErrsAndWarns"={0.0, 5.663716814159292, 7.168141592920354, 8.584070796460177}}, "ADAM3"={"Enbl"=FALSE, "ErrsAndWarns"={0.0, 5.663716814159292, 7.168141592920354, 8.584070796460177}}, "ADAM4"={"Enbl"=FALSE, "ErrsAndWarns"={0.0, 5.663716814159292, 7.168141592920354, 8.584070796460177}}, "72CoBeacFreq"={"Enbl"=FALSE, "ErrsAndWarns"={0.0, 5.663716814159292, 7.168141592920354, 8.584070796460177}}, "72CoCalFreq"={"Enbl"=FALSE, "ErrsAndWarns"={0.0, 5.663716814159292, 7.168141592920354, 8.584070796460177}}, "84CoBeacFreq"={"Enbl"=FALSE, "ErrsAndWarns"={0.0, 5.663716814159292, 7.168141592920354, 8.584070796460177}}, "84CoCalFreq"={"Enbl"=FALSE, "ErrsAndWarns"={0.0, 5.663716814159292, 7.168141592920354, 8.584070796460177}}, "72Co_CalTonePwr"={"Enbl"=FALSE, "ErrsAndWarns"={0.0, 5.663716814159292, 7.168141592920354, 8.584070796460177}}, "72X_CalTonePwr"={"Enbl"=FALSE, "ErrsAndWarns"={0.0, 5.663716814159292, 7.168141592920354, 8.584070796460177}}, "84Co_CalTonePwr"={"Enbl"=FALSE, "ErrsAndWarns"={0.0, 5.663716814159292, 7.168141592920354, 8.584070796460177}}, "84X_CalTonePwr"={"Enbl"=FALSE, "ErrsAndWarns"={0.0, 5.663716814159292, 7.168141592920354, 8.584070796460177}}}, "DO"=[], "AllAlarms"=[], "Alarm Status"={"Green"=FALSE, "Rx_Yell"=FALSE, "Cx_Yell"=FALSE, "Red"=FALSE, "Source"=""}, "SaturationStatus"={"84"=[], "72"=[]}, "WeatherStatus"=[], "10HzRefs"={"72Co_dset"=0, "84Co_dset"=0, "FileRef"=0}} {"10HzRefs"."FileRef" format="%.0x"; "10HzRefs"."84Co_dset" format="%.0x"; "10HzRefs"."72Co_dset" format="%.0x"; "AlarmCfg"."84X_CalTonePwr"."ErrsAndWarns" scale=-120.0..-45.0; "AlarmCfg"."72X_CalTonePwr"."ErrsAndWarns" scale=-120.0..-45.0; "AlarmCfg"."84Co_CalTonePwr"."ErrsAndWarns" scale=-120.0..-45.0; "AlarmCfg"."72Co_CalTonePwr"."ErrsAndWarns" scale=-120.0..-45.0; "AlarmCfg"."84CoCalFreq"."ErrsAndWarns" scale=24.9..25.1; "AlarmCfg"."84CoBeacFreq"."ErrsAndWarns" scale=25.5..27.0; "AlarmCfg"."72CoCalFreq"."ErrsAndWarns" scale=24.9..25.1; "AlarmCfg"."72CoBeacFreq"."ErrsAndWarns" scale=25.5..27.0; "AlarmCfg"."ADAM4"."ErrsAndWarns" scale=30.0..52.0; "AlarmCfg"."ADAM3"."ErrsAndWarns" scale=30.0..52.0; "AlarmCfg"."ADAM2"."ErrsAndWarns" scale=30.0..52.0; "AlarmCfg"."ADAM1"."ErrsAndWarns" scale=30.0..52.0; "AlarmCfg"."TE3"."ErrsAndWarns" scale=30.0..52.0; "AlarmCfg"."TE2"."ErrsAndWarns" scale=30.0..52.0; "AlarmCfg"."TE1"."ErrsAndWarns" scale=20.0..52.0; "AlarmCfg"."AI19"."ErrsAndWarns" scale=0.0..60.0; "AlarmCfg"."AI18"."ErrsAndWarns" scale=-10.0..10.0; "AlarmCfg"."AI6"."ErrsAndWarns" scale=0.0..35.0; "AlarmCfg"."AI5"."ErrsAndWarns" scale=0.0..20.0; "AlarmCfg"."AI4"."ErrsAndWarns" scale=0.0..15.0; "AlarmCfg"."AI3"."ErrsAndWarns" scale=0.0..10.0; "AlarmCfg"."AI2"."ErrsAndWarns" scale=0.0..10.0; "AlarmCfg"."TC13"."ErrsAndWarns" scale=-10.0..40.0; "LogData"."NoiseInfo"."HDF5_NoiseInfo"."Sum" format="%^#.1g"; "HDFRefs2"."Complex"."Group_ref" format="%.0x"; "HDFRefs2"."Complex"."QSpect_dset" format="%.0x"; "HDFRefs2"."Complex"."ISpect_dset" format="%.0x"; "HDFRefs2"."Complex"."PwrSpect_dset" format="%.0x"; "HDFRefs2"."Complex"."TImeStamp_dset" format="%.0x"; "HDFRefs2"."ADAM_Refs"."Group_ref" format="%.0x"; "HDFRefs2"."ADAM_Refs"."ADAM_CoPol_dset" format="%.0x"; "HDFRefs2"."ADAM_Refs"."ADAM_XPol_dset" format="%.0x"; "HDFRefs2"."ADAM_Refs"."ADAM_Noise_dset" format="%.0x"; "HDFRefs2"."ADAM_Refs"."ADAM_CalBox_dset" format="%.0x"; "HDFRefs2"."ADAM_Refs"."TimeStamp" format="%.0x"; "HDFRefs2"."Filter_Refs"."Filter_Group_ref" format="%.0x"; "HDFRefs2"."Filter_Refs"."TimeStamp_dset" format="%.0x"; "HDFRefs2"."Filter_Refs"."Filter_dset" format="%.0x"; "HDFRefs2"."AI_Refs"."BlowerPwr_dset" format="%.0x"; "HDFRefs2"."AI_Refs"."ElStdDev_dset" format="%.0x"; "HDFRefs2"."AI_Refs"."AzStdDev_dset" format="%.0x"; "HDFRefs2"."AI_Refs"."AI19_dset" format="%.0x"; "HDFRefs2"."AI_Refs"."AI18_dset" format="%.0x"; "HDFRefs2"."AI_Refs"."AI17_dset" format="%.0x"; "HDFRefs2"."AI_Refs"."AI16_dset" format="%.0x"; "HDFRefs2"."AI_Refs"."AI6_dset" format="%.0x"; "HDFRefs2"."AI_Refs"."AI5_dset" format="%.0x"; "HDFRefs2"."AI_Refs"."AI4_dset" format="%.0x"; "HDFRefs2"."AI_Refs"."AI3_dset" format="%.0x"; "HDFRefs2"."AI_Refs"."AI2_dset" format="%.0x"; "HDFRefs2"."AI_Refs"."AI0_dset" format="%.0x"; "HDFRefs2"."AI_Refs"."AI1_dset" format="%.0x"; "HDFRefs2"."AI_Refs"."TimeString_dset" format="%.0x"; "HDFRefs2"."AI_Refs"."TimeStamp_dset" format="%.0x"; "HDFRefs2"."AI_Refs"."Group_ref" format="%.0x"; "HDFRefs2"."Weath_Refs"."WindDirSTD_dset" format="%.0x"; "HDFRefs2"."Weath_Refs"."WindGusts_dset" format="%.0x"; "HDFRefs2"."Weath_Refs"."RainFall_dset" format="%.0x"; "HDFRefs2"."Weath_Refs"."RainRate_dset" format="%.0x"; "HDFRefs2"."Weath_Refs"."Pressure_dset" format="%.0x"; "HDFRefs2"."Weath_Refs"."Humidity_dset" format="%.0x"; "HDFRefs2"."Weath_Refs"."Temp_dset" format="%.0x"; "HDFRefs2"."Weath_Refs"."WindDir_dset" format="%.0x"; "HDFRefs2"."Weath_Refs"."WindSpd_dset" format="%.0x"; "HDFRefs2"."Weath_Refs"."TimeStamp_dset" format="%.0x"; "HDFRefs2"."Weath_Refs"."Group_ref" format="%.0x"; "HDFRefs2"."Weath_Refs"."TimeString_dset" format="%.0x"; "HDFRefs2"."UPS_Refs_Deprecated"."TimeStamp_dset" format="%.0x"; "HDFRefs2"."UPS_Refs_Deprecated"."TimeString_dset" format="%.0x"; "HDFRefs2"."UPS_Refs_Deprecated"."%_dset" format="%.0x"; "HDFRefs2"."UPS_Refs_Deprecated"."W_dset" format="%.0x"; "HDFRefs2"."UPS_Refs_Deprecated"."Hz_dset" format="%.0x"; "HDFRefs2"."UPS_Refs_Deprecated"."A_dset" format="%.0x"; "HDFRefs2"."UPS_Refs_Deprecated"."V_dset" format="%.0x"; "HDFRefs2"."UPS_Refs_Deprecated"."Group_ref" format="%.0x"; "HDFRefs2"."TE_Refs"."TimeStamp" format="%.0x"; "HDFRefs2"."TE_Refs"."TE_Outp3_dset" format="%.0x"; "HDFRefs2"."TE_Refs"."TE_Temp3_dset" format="%.0x"; "HDFRefs2"."TE_Refs"."TE_Outp2_dset" format="%.0x"; "HDFRefs2"."TE_Refs"."TE_Temp2_dset" format="%.0x"; "HDFRefs2"."TE_Refs"."TE_Outp1_dset" format="%.0x"; "HDFRefs2"."TE_Refs"."TE_Temp1_dset" format="%.0x"; "HDFRefs2"."TE_Refs"."Group_ref" format="%.0x"; "HDFRefs2"."DisdromRefs"."Status_dset_deprecated" format="%.0x"; "HDFRefs2"."DisdromRefs"."Spectrum_dset" format="%.0x"; "HDFRefs2"."DisdromRefs"."SpectGroup_ref" format="%.0x"; "HDFRefs2"."DisdromRefs"."HydromType_dset" format="%.0x"; "HDFRefs2"."DisdromRefs"."UnknownVolum_dset" format="%.0x"; "HDFRefs2"."DisdromRefs"."UnknownParticls_dset" format="%.0x"; "HDFRefs2"."DisdromRefs"."NonHydrVolum_dset" format="%.0x"; "HDFRefs2"."DisdromRefs"."NonHydrParticls_dset" format="%.0x"; "HDFRefs2"."DisdromRefs"."ParticlMinDiam_dset" format="%.0x"; "HDFRefs2"."DisdromRefs"."ParticlMaxSpeed_dset" format="%.0x"; "HDFRefs2"."DisdromRefs"."RadarReflect_dset" format="%.0x"; "HDFRefs2"."DisdromRefs"."Visibility_dset" format="%.0x"; "HDFRefs2"."DisdromRefs"."TotalRain_dset" format="%.0x"; "HDFRefs2"."DisdromRefs"."Solid_dset" format="%.0x"; "HDFRefs2"."DisdromRefs"."Liquid_dset" format="%.0x"; "HDFRefs2"."DisdromRefs"."TotalRainRate_dset" format="%.0x"; "HDFRefs2"."DisdromRefs"."TimeStamp_dset" format="%.0x"; "HDFRefs2"."DisdromRefs"."ParticlMinSpeed_dset" format="%.0x"; "HDFRefs2"."DisdromRefs"."MeasdParticles_dset" format="%.0x"; "HDFRefs2"."DisdromRefs"."MaxDiam_dset" format="%.0x"; "HDFRefs2"."DisdromRefs"."BasicGroup_ref" format="%.0x"; "HDFRefs2"."ValidRefs"."Alarm_Source_dset" format="%.0x"; "HDFRefs2"."ValidRefs"."Time_AlarmChange_dset" format="%.0x"; "HDFRefs2"."ValidRefs"."Time_Valid_dset" format="%.0x"; "HDFRefs2"."ValidRefs"."Alarm_Valid_dset" format="%.0x"; "HDFRefs2"."ValidRefs"."Saturat_dset" format="%.0x"; "HDFRefs2"."ValidRefs"."Group_ref" format="%.0x"; "HDFRefs2"."ValidRefs"."Weath_Valid_dset" format="%.0x"; "HDFRefs2"."ValidRefs"."Disdr_Valid_dset" format="%.0x"; "HDFRefs2"."TC_Refs"."TC13_Tamb_Inter" format="%.0x"; "HDFRefs2"."TC_Refs"."TC12_Gen_Exhaust" format="%.0x"; "HDFRefs2"."TC_Refs"."TC11_HVAC_Cond_Out" format="%.0x"; "HDFRefs2"."TC_Refs"."TC10_HVAC_Cond_In" format="%.0x"; "HDFRefs2"."TC_Refs"."TC9_LP2_Lo" format="%.0x"; "HDFRefs2"."TC_Refs"."TC8_LP2_LoMid" format="%.0x"; "HDFRefs2"."TC_Refs"."TC7_LP2_Mid" format="%.0x"; "HDFRefs2"."TC_Refs"."TC6_LP2_MidHi" format="%.0x"; "HDFRefs2"."TC_Refs"."TC5_LP2_Hi" format="%.0x"; "HDFRefs2"."TC_Refs"."TC4_LP1_Lo" format="%.0x"; "HDFRefs2"."TC_Refs"."TC3_LP1_LoMid" format="%.0x"; "HDFRefs2"."TC_Refs"."TC2_LP1_Mid" format="%.0x"; "HDFRefs2"."TC_Refs"."TC1_LP1_MidHi" format="%.0x"; "HDFRefs2"."TC_Refs"."TC0_LP1_Hi" format="%.0x"; "HDFRefs2"."TC_Refs"."TimeString_dset" format="%.0x"; "HDFRefs2"."TC_Refs"."TimeStamp_dset" format="%.0x"; "HDFRefs2"."TC_Refs"."Group_ref" format="%.0x"; "HDFRefs2"."NoiseRefs"."TimeStamp_df_dset" format="%.0x"; "HDFRefs2"."NoiseRefs"."sum_dset" format="%.0x"; "HDFRefs2"."NoiseRefs"."df_dset" format="%.0x"; "HDFRefs2"."NoiseRefs"."TimeStamp_dset" format="%.0x"; "HDFRefs2"."NoiseRefs"."SumdSpectrum_dset" format="%.0x"; "HDFRefs2"."NoiseRefs"."TimeString_dset" format="%.0x"; "HDFRefs2"."NoiseRefs"."Group_ref" format="%.0x"; "HDFRefs2"."ToneRefs"."Group_ref" format="%.0x"; "HDFRefs2"."ToneRefs"."Cal"."Downshift_dset" format="%.0x"; "HDFRefs2"."ToneRefs"."Cal"."DeltaPhase_dset" format="%.0x"; "HDFRefs2"."ToneRefs"."Cal"."Phase_dset" format="%.0x"; "HDFRefs2"."ToneRefs"."Cal"."SNR_dset" format="%.0x"; "HDFRefs2"."ToneRefs"."Cal"."df_dset" format="%.0x"; "HDFRefs2"."ToneRefs"."Cal"."PeakLoc_dset" format="%.0x"; "HDFRefs2"."ToneRefs"."Cal"."MaxValue_dset" format="%.0x"; "HDFRefs2"."ToneRefs"."Cal"."TImeStamp_dset" format="%.0x"; "HDFRefs2"."ToneRefs"."Cal"."TimeString_dset" format="%.0x"; "HDFRefs2"."ToneRefs"."Beac"."Downshift_dset" format="%.0x"; "HDFRefs2"."ToneRefs"."Beac"."DeltaPhase_dset" format="%.0x"; "HDFRefs2"."ToneRefs"."Beac"."Phase_dset" format="%.0x"; "HDFRefs2"."ToneRefs"."Beac"."SNR_dset" format="%.0x"; "HDFRefs2"."ToneRefs"."Beac"."df_dset" format="%.0x"; "HDFRefs2"."ToneRefs"."Beac"."PeakLoc_dset" format="%.0x"; "HDFRefs2"."ToneRefs"."Beac"."MaxValue_dset" format="%.0x"; "HDFRefs2"."ToneRefs"."Beac"."TImeStamp_dset" format="%.0x"; "HDFRefs2"."ToneRefs"."Beac"."TimeString_dset" format="%.0x"; "HDFRefs2"."ToneRefs"."CalZoom_dSet" format="%.0x"; "HDFRefs2"."ToneRefs"."BeacZoom_dSet" format="%.0x"; "HDFRefs2"."File" format="%.0x"; "HDFRefs1"."Complex"."Group_ref" format="%.0x"; "HDFRefs1"."Complex"."QSpect_dset" format="%.0x"; "HDFRefs1"."Complex"."ISpect_dset" format="%.0x"; "HDFRefs1"."Complex"."PwrSpect_dset" format="%.0x"; "HDFRefs1"."Complex"."TImeStamp_dset" format="%.0x"; "HDFRefs1"."ADAM_Refs"."Group_ref" format="%.0x"; "HDFRefs1"."ADAM_Refs"."ADAM_CoPol_dset" format="%.0x"; "HDFRefs1"."ADAM_Refs"."ADAM_XPol_dset" format="%.0x"; "HDFRefs1"."ADAM_Refs"."ADAM_Noise_dset" format="%.0x"; "HDFRefs1"."ADAM_Refs"."ADAM_CalBox_dset" format="%.0x"; "HDFRefs1"."ADAM_Refs"."TimeStamp" format="%.0x"; "HDFRefs1"."Filter_Refs"."Filter_Group_ref" format="%.0x"; "HDFRefs1"."Filter_Refs"."TimeStamp_dset" format="%.0x"; "HDFRefs1"."Filter_Refs"."Filter_dset" format="%.0x"; "HDFRefs1"."AI_Refs"."BlowerPwr_dset" format="%.0x"; "HDFRefs1"."AI_Refs"."ElStdDev_dset" format="%.0x"; "HDFRefs1"."AI_Refs"."AzStdDev_dset" format="%.0x"; "HDFRefs1"."AI_Refs"."AI19_dset" format="%.0x"; "HDFRefs1"."AI_Refs"."AI18_dset" format="%.0x"; "HDFRefs1"."AI_Refs"."AI17_dset" format="%.0x"; "HDFRefs1"."AI_Refs"."AI16_dset" format="%.0x"; "HDFRefs1"."AI_Refs"."AI6_dset" format="%.0x"; "HDFRefs1"."AI_Refs"."AI5_dset" format="%.0x"; "HDFRefs1"."AI_Refs"."AI4_dset" format="%.0x"; "HDFRefs1"."AI_Refs"."AI3_dset" format="%.0x"; "HDFRefs1"."AI_Refs"."AI2_dset" format="%.0x"; "HDFRefs1"."AI_Refs"."AI0_dset" format="%.0x"; "HDFRefs1"."AI_Refs"."AI1_dset" format="%.0x"; "HDFRefs1"."AI_Refs"."TimeString_dset" format="%.0x"; "HDFRefs1"."AI_Refs"."TimeStamp_dset" format="%.0x"; "HDFRefs1"."AI_Refs"."Group_ref" format="%.0x"; "HDFRefs1"."Weath_Refs"."WindDirSTD_dset" format="%.0x"; "HDFRefs1"."Weath_Refs"."WindGusts_dset" format="%.0x"; "HDFRefs1"."Weath_Refs"."RainFall_dset" format="%.0x"; "HDFRefs1"."Weath_Refs"."RainRate_dset" format="%.0x"; "HDFRefs1"."Weath_Refs"."Pressure_dset" format="%.0x"; "HDFRefs1"."Weath_Refs"."Humidity_dset" format="%.0x"; "HDFRefs1"."Weath_Refs"."Temp_dset" format="%.0x"; "HDFRefs1"."Weath_Refs"."WindDir_dset" format="%.0x"; "HDFRefs1"."Weath_Refs"."WindSpd_dset" format="%.0x"; "HDFRefs1"."Weath_Refs"."TimeStamp_dset" format="%.0x"; "HDFRefs1"."Weath_Refs"."Group_ref" format="%.0x"; "HDFRefs1"."Weath_Refs"."TimeString_dset" format="%.0x"; "HDFRefs1"."UPS_Refs_Deprecated"."TimeStamp_dset" format="%.0x"; "HDFRefs1"."UPS_Refs_Deprecated"."TimeString_dset" format="%.0x"; "HDFRefs1"."UPS_Refs_Deprecated"."%_dset" format="%.0x"; "HDFRefs1"."UPS_Refs_Deprecated"."W_dset" format="%.0x"; "HDFRefs1"."UPS_Refs_Deprecated"."Hz_dset" format="%.0x"; "HDFRefs1"."UPS_Refs_Deprecated"."A_dset" format="%.0x"; "HDFRefs1"."UPS_Refs_Deprecated"."V_dset" format="%.0x"; "HDFRefs1"."UPS_Refs_Deprecated"."Group_ref" format="%.0x"; "HDFRefs1"."TE_Refs"."TimeStamp" format="%.0x"; "HDFRefs1"."TE_Refs"."TE_Outp3_dset" format="%.0x"; "HDFRefs1"."TE_Refs"."TE_Temp3_dset" format="%.0x"; "HDFRefs1"."TE_Refs"."TE_Outp2_dset" format="%.0x"; "HDFRefs1"."TE_Refs"."TE_Temp2_dset" format="%.0x"; "HDFRefs1"."TE_Refs"."TE_Outp1_dset" format="%.0x"; "HDFRefs1"."TE_Refs"."TE_Temp1_dset" format="%.0x"; "HDFRefs1"."TE_Refs"."Group_ref" format="%.0x"; "HDFRefs1"."DisdromRefs"."Status_dset_deprecated" format="%.0x"; "HDFRefs1"."DisdromRefs"."Spectrum_dset" format="%.0x"; "HDFRefs1"."DisdromRefs"."SpectGroup_ref" format="%.0x"; "HDFRefs1"."DisdromRefs"."HydromType_dset" format="%.0x"; "HDFRefs1"."DisdromRefs"."UnknownVolum_dset" format="%.0x"; "HDFRefs1"."DisdromRefs"."UnknownParticls_dset" format="%.0x"; "HDFRefs1"."DisdromRefs"."NonHydrVolum_dset" format="%.0x"; "HDFRefs1"."DisdromRefs"."NonHydrParticls_dset" format="%.0x"; "HDFRefs1"."DisdromRefs"."ParticlMinDiam_dset" format="%.0x"; "HDFRefs1"."DisdromRefs"."ParticlMaxSpeed_dset" format="%.0x"; "HDFRefs1"."DisdromRefs"."RadarReflect_dset" format="%.0x"; "HDFRefs1"."DisdromRefs"."Visibility_dset" format="%.0x"; "HDFRefs1"."DisdromRefs"."TotalRain_dset" format="%.0x"; "HDFRefs1"."DisdromRefs"."Solid_dset" format="%.0x"; "HDFRefs1"."DisdromRefs"."Liquid_dset" format="%.0x"; "HDFRefs1"."DisdromRefs"."TotalRainRate_dset" format="%.0x"; "HDFRefs1"."DisdromRefs"."TimeStamp_dset" format="%.0x"; "HDFRefs1"."DisdromRefs"."ParticlMinSpeed_dset" format="%.0x"; "HDFRefs1"."DisdromRefs"."MeasdParticles_dset" format="%.0x"; "HDFRefs1"."DisdromRefs"."MaxDiam_dset" format="%.0x"; "HDFRefs1"."DisdromRefs"."BasicGroup_ref" format="%.0x"; "HDFRefs1"."ValidRefs"."Alarm_Source_dset" format="%.0x"; "HDFRefs1"."ValidRefs"."Time_AlarmChange_dset" format="%.0x"; "HDFRefs1"."ValidRefs"."Time_Valid_dset" format="%.0x"; "HDFRefs1"."ValidRefs"."Alarm_Valid_dset" format="%.0x"; "HDFRefs1"."ValidRefs"."Saturat_dset" format="%.0x"; "HDFRefs1"."ValidRefs"."Group_ref" format="%.0x"; "HDFRefs1"."ValidRefs"."Weath_Valid_dset" format="%.0x"; "HDFRefs1"."ValidRefs"."Disdr_Valid_dset" format="%.0x"; "HDFRefs1"."TC_Refs"."TC13_Tamb_Inter" format="%.0x"; "HDFRefs1"."TC_Refs"."TC12_Gen_Exhaust" format="%.0x"; "HDFRefs1"."TC_Refs"."TC11_HVAC_Cond_Out" format="%.0x"; "HDFRefs1"."TC_Refs"."TC10_HVAC_Cond_In" format="%.0x"; "HDFRefs1"."TC_Refs"."TC9_LP2_Lo" format="%.0x"; "HDFRefs1"."TC_Refs"."TC8_LP2_LoMid" format="%.0x"; "HDFRefs1"."TC_Refs"."TC7_LP2_Mid" format="%.0x"; "HDFRefs1"."TC_Refs"."TC6_LP2_MidHi" format="%.0x"; "HDFRefs1"."TC_Refs"."TC5_LP2_Hi" format="%.0x"; "HDFRefs1"."TC_Refs"."TC4_LP1_Lo" format="%.0x"; "HDFRefs1"."TC_Refs"."TC3_LP1_LoMid" format="%.0x"; "HDFRefs1"."TC_Refs"."TC2_LP1_Mid" format="%.0x"; "HDFRefs1"."TC_Refs"."TC1_LP1_MidHi" format="%.0x"; "HDFRefs1"."TC_Refs"."TC0_LP1_Hi" format="%.0x"; "HDFRefs1"."TC_Refs"."TimeString_dset" format="%.0x"; "HDFRefs1"."TC_Refs"."TimeStamp_dset" format="%.0x"; "HDFRefs1"."TC_Refs"."Group_ref" format="%.0x"; "HDFRefs1"."NoiseRefs"."TimeStamp_df_dset" format="%.0x"; "HDFRefs1"."NoiseRefs"."sum_dset" format="%.0x"; "HDFRefs1"."NoiseRefs"."df_dset" format="%.0x"; "HDFRefs1"."NoiseRefs"."TimeStamp_dset" format="%.0x"; "HDFRefs1"."NoiseRefs"."SumdSpectrum_dset" format="%.0x"; "HDFRefs1"."NoiseRefs"."TimeString_dset" format="%.0x"; "HDFRefs1"."NoiseRefs"."Group_ref" format="%.0x"; "HDFRefs1"."ToneRefs"."Group_ref" format="%.0x"; "HDFRefs1"."ToneRefs"."Cal"."Downshift_dset" format="%.0x"; "HDFRefs1"."ToneRefs"."Cal"."DeltaPhase_dset" format="%.0x"; "HDFRefs1"."ToneRefs"."Cal"."Phase_dset" format="%.0x"; "HDFRefs1"."ToneRefs"."Cal"."SNR_dset" format="%.0x"; "HDFRefs1"."ToneRefs"."Cal"."df_dset" format="%.0x"; "HDFRefs1"."ToneRefs"."Cal"."PeakLoc_dset" format="%.0x"; "HDFRefs1"."ToneRefs"."Cal"."MaxValue_dset" format="%.0x"; "HDFRefs1"."ToneRefs"."Cal"."TImeStamp_dset" format="%.0x"; "HDFRefs1"."ToneRefs"."Cal"."TimeString_dset" format="%.0x"; "HDFRefs1"."ToneRefs"."Beac"."Downshift_dset" format="%.0x"; "HDFRefs1"."ToneRefs"."Beac"."DeltaPhase_dset" format="%.0x"; "HDFRefs1"."ToneRefs"."Beac"."Phase_dset" format="%.0x"; "HDFRefs1"."ToneRefs"."Beac"."SNR_dset" format="%.0x"; "HDFRefs1"."ToneRefs"."Beac"."df_dset" format="%.0x"; "HDFRefs1"."ToneRefs"."Beac"."PeakLoc_dset" format="%.0x"; "HDFRefs1"."ToneRefs"."Beac"."MaxValue_dset" format="%.0x"; "HDFRefs1"."ToneRefs"."Beac"."TImeStamp_dset" format="%.0x"; "HDFRefs1"."ToneRefs"."Beac"."TimeString_dset" format="%.0x"; "HDFRefs1"."ToneRefs"."CalZoom_dSet" format="%.0x"; "HDFRefs1"."ToneRefs"."BeacZoom_dSet" format="%.0x"; "HDFRefs1"."File" format="%.0x"; "Config"."FP_User"."Deadband" format="%#.0f"}, 7 "10 Hz file ref":T1 format="%.0x")   [LabVIEW 2018]
doc: "Creates a file path for the data log and for the redundant data log. \nOpens both files and returns: \n*File References\n*Boolean Status: File already exists"
uses:
  Controls/Clusts/LogLoopClust.ctl
  Controls/Clusts/Config_Clust.ctl
  Controls/Clusts/UserConfig.ctl
  Controls/PathsCluster.ctl
  Controls/Clusts/FrontPanel_UserConfig.ctl
  Controls/Clusts/Inclinometer_User_Cfg.ctl
  Controls/Clusts/FP_UserTargetConfig.ctl
  Controls/Clusts/FreqShift.ctl
  Controls/Clusts/FPGA_Scale.ctl
  Controls/Enums/ScaleMeasure.ctl
  Controls/RadioButtons/FilterEnableRadio.ctl
  Controls/Enums/TargetNumber.ctl
  Controls/Clusts/HDF5_File_Refs.ctl
  <vilib>/addons/h5labview2/base/hid_t.ctl
  Controls/Clusts/ToneGroupRefsClust.ctl
  HDF5/HDF5_Tone_refs.ctl
  HDF5/HDF5_Noise_refs.ctl
  HDF5/TC_Tone_refs.ctl
  HDF5/HDF5_Validty_refs.ctl
  HDF5/HDF5_Disdrometer_Refs.ctl
  HDF5/HDF5_Health_Refs.ctl
  HDF5/UPS_refs.ctl
  Controls/Clusts/WeatherRefs.ctl
  HDF5/HDF5_AI_refs.ctl
  HDF5/HDF5_Filter_refs.ctl
  HDF5/HDF5_ADAM_Refs.ctl
  HDF5/HDF5_Complex_Refs.ctl
  Controls/Clusts/LogDataClust.ctl
  Controls/Clusts/ToneLogBuffered.ctl
  Controls/Clusts/SaturationMonitorBuffer.ctl
  HDF5/TC_Data_Structure.ctl
  Controls/Clusts/AI_Clust.ctl
  HDF5/HDF5_NoiseInfoClust.ctl
  HDF5/DisdrometerData.ctl
  HDF5/DisdromterSummaryData.ctl
  Disdrometer/Disdrometer_Status_Cluster.ctl
  Controls/Clusts/WeatherDataClust.ctl
  Controls/Clusts/ValidityWeatherClust.ctl
  Controls/Clusts/TE_Data_Clust.ctl
  HDF5/HDF5_ADAM_Data.ctl
  Controls/Clusts/TimeDomainData.ctl
  Controls/Clusts/AlarmSettingsClust.ctl
  Controls/Clusts/AlarmThresh_OneChan.ctl
  Controls/Clusts/ErrorStatus.ctl
  Controls/Clusts/DigOutClust.ctl
  Controls/Clusts/Saturation_Status_Clust.ctl
  Controls/Clusts/HDF5_10HzRefs.ctl
  <vilib>/addons/h5labview2/file/H5Fmode.ctl
  <vilib>/addons/h5labview2/file/H5F.lvlib
types:
  T1 = typedef "hid_t.ctl" = i32
  T2 = typedef "LogLoopClust.ctl" = cluster{"base path":path, "PathNow1":path, "PathNow2":path, "DateNow":string, "NAS path":path, "LogFiltStage":bool, "LogNoise_df_1":bool, "LogNoise_df_2":bool, "LogNoise_df_3":bool, "LogNoise_df_4":bool, "Config":T3, "HDFRefs1":T14, "HDFRefs2":T14, "LogData":T28, "AlarmCfg":T42, "DO":bool[], "AllAlarms":T44[], "Alarm Status":T45, "SaturationStatus":T46, "WeatherStatus":bool[], "10HzRefs":T47}
  T3 = typedef "Config_Clust.ctl" = cluster{"UsrCfg":T4, "FP_User":T6}
  T4 = typedef "UserConfig.ctl" = cluster{"Paths":T5, "SampleRate":dbl}
  T5 = typedef "PathsCluster.ctl" = cluster{"CfgFile":path, "LogFolder":path, "LogFile":path, "NAS path":path, "ThreshFile":path, "RedunFolder":path}
  T6 = typedef "FrontPanel_UserConfig.ctl" = cluster{"#NoiseSums":u32, "Max_df":u32, "AvgAvg":bool, "#Avg":u16, "AutoCenter":bool, "Inclin":T7, "1":T8, "2":T8, "3":T8, "4":T8, "Target to Probe":T13, "SNR_Thresh":dbl, "Paths":T5, "Connex_Location":string, "SimulateFPGA":bool, "Deadband":dbl}
  T7 = typedef "Inclinometer_User_Cfg.ctl" = cluster{"Vmin":dbl, "Vmax":dbl, "Angle_min":dbl, "Angle_max":dbl, "Offset":dbl, "Pos_Neg":bool}
  T8 = typedef "FP_UserTargetConfig.ctl" = cluster{"Cal_":T9, "Beac":T9, "Scale":T10, "Offset":fxp<+/-,16,16>, "Scale_Noise":fxp<+/-,30,30>, "Scale_Step1":fxp<+/-,17,17>, "Scale_In_RT":ext, "ScaleMeas":fxp<+/-,16,1>, "FreqsToRemove":i32[], "Width":i32[], "ScaleMeasEnum":T11, "FilterEnab":T12}
  T9 = typedef "FreqShift.ctl" = cluster{"Fine":dbl, "Coarse_":dbl}
  T10 = typedef "FPGA_Scale.ctl" = cluster{"Step4":fxp<+/-,23,23>, "Step5":fxp<+/-,23,23>, "Step6":fxp<+/-,23,23>, "Step7":fxp<+/-,23,23>}
  T11 = typedef "ScaleMeasure.ctl" = enum16{"1", "10", "50", "42"}
  T12 = typedef "FilterEnableRadio.ctl" = enum32{"None", "Step 1", "Frequency Shift", "Step 4", "Step 5", "Step 6", "Step 7"}
  T13 = typedef "TargetNumber.ctl" = enum16{"1", "2", "3", "4"}
  T14 = typedef "HDF5_File_Refs.ctl" = cluster{"File":T1, "ToneRefs":T15[], "NoiseRefs":T17[], "TC_Refs":T18, "ValidRefs":T19, "DisdromRefs":T20, "TE_Refs":T21, "UPS_Refs_Deprecated":T22, "Weath_Refs":T23, "AI_Refs":T24, "Filter_Refs":T25, "ADAM_Refs":T26, "Complex":T27[]}
  T15 = typedef "ToneGroupRefsClust.ctl" = cluster{"Group_ref":T1, "Cal":T16, "Beac":T16, "CalZoom_dSet":T1, "BeacZoom_dSet":T1}
  T16 = typedef "HDF5_Tone_refs.ctl" = cluster{"TimeString_dset":T1, "TImeStamp_dset":T1, "SNR_dset":T1, "MaxValue_dset":T1, "PeakLoc_dset":T1, "df_dset":T1, "Phase_dset":T1, "DeltaPhase_dset":T1, "Downshift_dset":T1}
  T17 = typedef "HDF5_Noise_refs.ctl" = cluster{"Group_ref":T1, "TimeString_dset":T1, "TimeStamp_dset":T1, "TimeStamp_df_dset":T1, "df_dset":T1, "sum_dset":T1, "SumdSpectrum_dset":T1}
  T18 = typedef "TC_Tone_refs.ctl" = cluster{"Group_ref":T1, "TimeString_dset":T1, "TimeStamp_dset":T1, "TC0_LP1_Hi":T1, "TC1_LP1_MidHi":T1, "TC2_LP1_Mid":T1, "TC3_LP1_LoMid":T1, "TC4_LP1_Lo":T1, "TC5_LP2_Hi":T1, "TC6_LP2_MidHi":T1, "TC7_LP2_Mid":T1, "TC8_LP2_LoMid":T1, "TC9_LP2_Lo":T1, "TC10_HVAC_Cond_In":T1, "TC11_HVAC_Cond_Out":T1, "TC12_Gen_Exhaust":T1, "TC13_Tamb_Inter":T1}
  T19 = typedef "HDF5_Validty_refs.ctl" = cluster{"Group_ref":T1, "Weath_Valid_dset":T1, "Disdr_Valid_dset":T1, "Saturat_dset":T1, "Alarm_Valid_dset":T1, "Time_Valid_dset":T1, "Time_AlarmChange_dset":T1, "Alarm_Source_dset":T1}
  T20 = typedef "HDF5_Disdrometer_Refs.ctl" = cluster{"BasicGroup_ref":T1, "TimeStamp_dset":T1, "TotalRainRate_dset":T1, "Liquid_dset":T1, "Solid_dset":T1, "TotalRain_dset":T1, "Visibility_dset":T1, "RadarReflect_dset":T1, "MaxDiam_dset":T1, "MeasdParticles_dset":T1, "ParticlMinSpeed_dset":T1, "ParticlMaxSpeed_dset":T1, "ParticlMinDiam_dset":T1, "NonHydrParticls_dset":T1, "NonHydrVolum_dset":T1, "UnknownParticls_dset":T1, "UnknownVolum_dset":T1, "HydromType_dset":T1, "SpectGroup_ref":T1, "Spectrum_dset":T1, "Status_dset_deprecated":T1}
  T21 = typedef "HDF5_Health_Refs.ctl" = cluster{"Group_ref":T1, "TE_Temp1_dset":T1, "TE_Outp1_dset":T1, "TE_Temp2_dset":T1, "TE_Outp2_dset":T1, "TE_Temp3_dset":T1, "TE_Outp3_dset":T1, "TimeStamp":T1}
  T22 = typedef "UPS_refs.ctl" = cluster{"Group_ref":T1, "TimeString_dset":T1, "TimeStamp_dset":T1, "V_dset":T1, "A_dset":T1, "Hz_dset":T1, "W_dset":T1, "%_dset":T1}
  T23 = typedef "WeatherRefs.ctl" = cluster{"Group_ref":T1, "TimeString_dset":T1, "TimeStamp_dset ":T1, "WindSpd_dset":T1, "WindGusts_dset":T1, "WindDir_dset":T1, "WindDirSTD_dset":T1, "Temp_dset":T1, "Humidity_dset":T1, "Pressure_dset":T1, "RainRate_dset":T1, "RainFall_dset":T1}
  T24 = typedef "HDF5_AI_refs.ctl" = cluster{"Group_ref":T1, "TimeString_dset":T1, "TimeStamp_dset":T1, "AI0_dset":T1, "AI1_dset":T1, "AI2_dset":T1, "AI3_dset":T1, "AI4_dset":T1, "AI5_dset":T1, "AI6_dset":T1, "AI16_dset":T1, "AI17_dset":T1, "AI18_dset":T1, "AzStdDev_dset":T1, "AI19_dset":T1, "ElStdDev_dset":T1, "BlowerPwr_dset":T1}
  T25 = typedef "HDF5_Filter_refs.ctl" = cluster{"Filter_Group_ref":T1, "TimeStamp_dset":T1, "Filter_dset":T1}
  T26 = typedef "HDF5_ADAM_Refs.ctl" = cluster{"Group_ref":T1, "ADAM_CoPol_dset":T1, "ADAM_XPol_dset":T1, "ADAM_Noise_dset":T1, "ADAM_CalBox_dset":T1, "TimeStamp":T1}
  T27 = typedef "HDF5_Complex_Refs.ctl" = cluster{"Group_ref":T1, "TImeStamp_dset":T1, "PwrSpect_dset":T1, "ISpect_dset":T1, "QSpect_dset":T1}
  T28 = typedef "LogDataClust.ctl" = cluster{"Tone":T29[], "TCData":T31, "AI":T32, "NoiseTrace":cluster{"Target":T13, "NoiseTrace":dbl[]}[], "NoiseInfo":cluster{"Target":T13, "HDF5_NoiseInfo":T33}[], "Disdrom":T34[], "Weath":T37[], "TE":T39, "ADAM":T40, "TimeDomain":T41[]}
  T29 = typedef "ToneLogBuffered.ctl" = cluster{"Count":i32, "CalVal":sgl[], "CalLoc":i32[], "BeacVal":sgl[], "BeacLoc":i32[], "BeacShift":i32[], "Enum":T13, "df":dbl, "PwrSpectr":sgl[][], "ISpectr":sgl[][], "QSpectr":sgl[][], "Time":timestamp[], "SNR":sgl[], "AboveThresh":bool[], "10Hz_PeakVal":dbl[], "Phase":sgl[], "DeltaPhase":dbl[], "Saturat":T30, "10MHz":bool}
  T30 = typedef "SaturationMonitorBuffer.ctl" = cluster{"Meas":bool[], "Stage1":bool[], "Stage4":bool[], "Stage5":bool[], "Stage6":bool[], "Stage7":bool[]}
  T31 = typedef "TC_Data_Structure.ctl" = cluster{"TimeStamp":dbl, "TimeString":string, "TC0_LP1_Hi":dbl, "TC1_LP1_MidHi":dbl, "TC2_LP1_Mid":dbl, "TC3_LP1_LoMid":dbl, "TC4_LP1_Lo":dbl, "TC5_LP2_Hi":dbl, "TC6_LP2_MidHi":dbl, "TC7_LP2_Mid":dbl, "TC8_LP2_LoMid":dbl, "TC9_LP2_Lo":dbl, "TC10_HVAC_Cond_In":dbl, "TC11_HVAC_Cond_Out":dbl, "TC12_Gen_Exhaust":dbl, "TC13_Amb_Inter":dbl, "TC14_Unused":dbl, "TC15_Unused":dbl, "TC16_Unused":dbl, "TC17_Unused":dbl, "TC18_Unused":dbl, "TC19_Unused":dbl, "TC20_Unused":dbl, "TC21_Unused":dbl, "TC22_Unused":dbl, "TC23_Unused":dbl, "TC24_Unused":dbl, "TC25_Unused":dbl, "TC26_Unused":dbl, "TC27_Unused":dbl, "TC28_Unused":dbl, "TC29_Unused":dbl, "TC30_Unused":dbl, "TC31_Unused":dbl}
  T32 = typedef "AI_Clust.ctl" = cluster{"TimeString":string, "Time Stamp":dbl, "AI0_Unused":dbl, "AI1_-5V":dbl, "AI2_+5V":dbl, "AI3_+6V":dbl, "AI4_+12V":dbl, "AI5_+15V":dbl, "AI6_+28V":dbl, "AI7_Unused":dbl, "Ai16_72GHz_CalPower":dbl, "Ai17_84GHz_CalPower":dbl, "Ai18_InclinAz":dbl, "Ai19_InclinEl":dbl, "Ai20_BlowerPwr":dbl, "Ai21_Unused":dbl, "Ai22_Unused":dbl, "Ai23_Unused":dbl, "InclinA_StdDev":dbl, "InclinB_StdDev":dbl, "InclinAz_Unfilt":dbl, "InclinEl_Unfilt":dbl}
  T33 = typedef "HDF5_NoiseInfoClust.ctl" = cluster{"Timestring":string, "Timestamp":dbl, "df":dbl, "Sum":dbl}
  T34 = typedef "DisdrometerData.ctl" = cluster{"Spectrum Data":i16[], "DisdromSummary":T35, "Status":T36}
  T35 = typedef "DisdromterSummaryData.ctl" = cluster{"current time":dbl, "Timestamp":dbl, "Total Rain Rate":dbl, "Liquid Rain Rate":dbl, "Solid Rain Rate":dbl, "Total Rainfall":dbl, "Visibility":dbl, "Radar Reflectivity":dbl, "Max Diameter Hail":dbl, "Measured Particles":i32, "Particle Min Speed":i16, "Particle Max Speed":i16, "Particle Min Diam":i16, "NonHydr Particles":i16, "NonHydr Volume":dbl, "Unkn Particles":i16, "Unkn Volume":dbl, "HydroType":i8}
  T36 = typedef "Disdrometer_Status_Cluster.ctl" = cluster{"Laser":bool, "Signal":bool, "LaserTemp_Analog":bool, "LaserTemp_Digital":bool, "LaserCurrent_Analog":bool, "LaserCurrent_Digital":bool, "SensorSupply":bool, "HeatLaserHead":bool, "HeatReceiverHead":bool, "TempSensor":bool, "HeatSupply":bool, "HeatHousing":bool, "HeatHeads":bool, "HeatCarriers":bool, "OutputLaserPower":bool, "Checksum":bool, "StatusInt":u16}
  T37 = typedef "WeatherDataClust.ctl" = cluster{"TimeString":string, "Timestamp":dbl, "Wind Speed":sgl, "Wind Gusts":sgl, "Wind Dir":sgl, "Wind Dir STD":sgl, "Temperature":sgl, "Humidity":sgl, "Pressure":sgl, "Rain Rate":i16, "Rain Fall":sgl, "Status":T38}
  T38 = typedef "ValidityWeatherClust.ctl" = cluster{"Temp_OutOfBounds":bool, "Temp_IncrSTD":bool, "Temp_Oth":bool, "BarPress_OutOfBounds":bool, "BarPress_IncrSTD":bool, "BarPress_Change":bool, "BarPress_Other":bool, "Humid_OutOfBounds":bool, "Humid_IncrSTD":bool, "Humid_Other":bool, "Wind__Spd_OutOfBounds":bool, "Wind_Dir_OutOfBounds":bool, "RainBuck_OutOfBounds":bool, "RainBuck_Disdrom":bool, "Disdrom_RainBuck":bool, "Placeholder":bool}
  T39 = typedef "TE_Data_Clust.ctl" = cluster{"TimeString":string, "TimeStamp":dbl, "Temp":dbl, "Output":dbl, "Temp 2":dbl, "Output 2":dbl, "Temp 3":dbl, "Output 3":dbl}
  T40 = typedef "HDF5_ADAM_Data.ctl" = cluster{"Timestamp":dbl, "Time string":string, "Fault 1":bool, "Fault 2":bool, "Fault 3":bool, "Fault 4":bool, "Fault 5":bool, "Fault 6":bool, "Value 1":dbl, "Value 2":dbl, "Value 3":dbl, "Value 4":dbl, "Value 5":dbl, "Value 6":dbl}
  T41 = typedef "TimeDomainData.ctl" = cluster{"CalTimeVal":dbl[], "CalTimeCount":u32[], "Enum":T13}
  T42 = typedef "AlarmSettingsClust.ctl" = cluster{"TC13":T43, "AI1":T43, "AI2":T43, "AI3":T43, "AI4":T43, "AI5":T43, "AI6":T43, "AI18":T43, "AI19":T43, "TE1":T43, "TE2":T43, "TE3":T43, "ADAM1":T43, "ADAM2":T43, "ADAM3":T43, "ADAM4":T43, "72CoBeacFreq":T43, "72CoCalFreq":T43, "84CoBeacFreq":T43, "84CoCalFreq":T43, "72Co_CalTonePwr":T43, "72X_CalTonePwr":T43, "84Co_CalTonePwr":T43, "84X_CalTonePwr":T43}
  T43 = typedef "AlarmThresh_OneChan.ctl" = cluster{"Enbl":bool, "ErrsAndWarns":cluster{dbl, dbl, dbl, dbl}}
  T44 = typedef "ErrorStatus.ctl" = cluster{"RX?":bool, "Warn":bool, "Error":bool, "Enabl":bool, "Source":string}
  T45 = typedef "DigOutClust.ctl" = cluster{"Green":bool, "Rx_Yell":bool, "Cx_Yell":bool, "Red":bool, "Source":string}
  T46 = typedef "Saturation_Status_Clust.ctl" = cluster{"84":bool[], "72":bool[]}
  T47 = typedef "HDF5_10HzRefs.ctl" = cluster{"72Co_dset":T1, "84Co_dset":T1, "FileRef":T1}
  T48 = typedef "H5F.lvlib/H5Fmode.ctl" = enum16{"read-only", "read-write", "overwrite", "create new", "open or create"}
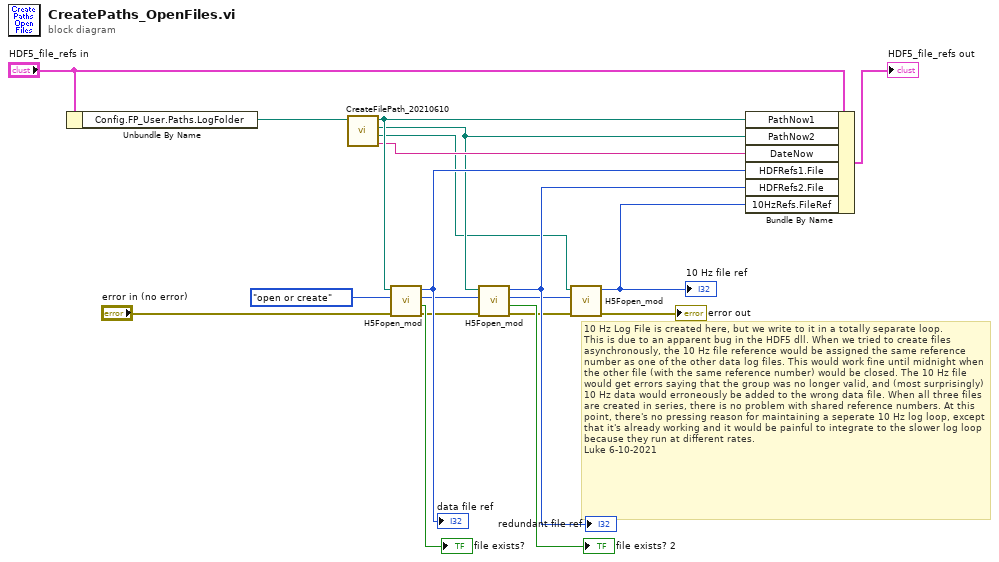
[diagram p0: block diagram]
diagram:
  w6 = H5Fmode."open or create" ("mode (read-only)")
  # "10 Hz Log File is created here, but we write to it in a totally separate loop.\nThis is due to an apparent bug in the HDF5 dll. When we tried to create files asynchronously, the 10 Hz file reference would be assigned the same reference number as one of the other data log files. This would work fine until midnight when the other file (with the same reference number) would be closed. The 10 Hz file would get errors saying that the group was no longer valid, and (most surprisingly) 10 Hz data would erroneously be added to the wrong data file. When all three files are created in series, there is no problem with shared reference numbers. At this point, there's no pressing reason for maintaining a seperate 10 Hz log loop, except that it's already working and it would be painful to integrate to the slower log loop because they run at different rates.\nLuke 6-10-2021"
  n1 = Unbundle By Name("HDF5_file_refs in") -> ("Config.FP_User.Paths.LogFolder"=w5:path)
  n2 = call "CreateFilePath_20210610.vi"("base path"=w5) -> ("DateString"=w4:string, "10 Hz appended path"=w2:path, "appended path 2"=w3:path, "appended path"=w10:path)  [unwired: 6 in, 1 out]
  n3 = call "H5Fopen_mod.vi"("error in (no error)"="error in (no error)", "mode (read-only)"=w6, "path"=w10) -> ("error out"=w9:errorcluster, "file exists?"=→"file exists?":bool, "ref out"=w15:T1)  [unwired: 6 in]
  "data file ref" <- w15
  n4 = call "H5Fopen_mod.vi"("error in (no error)"=w9, "mode (read-only)"=w6, "path"=w3) -> ("error out"=w8:errorcluster, "file exists?"=→"file exists? 2":bool, "ref out"=w13:T1)  [unwired: 6 in]
  "redundant file ref" <- w13
  n5 = call "H5Fopen_mod.vi"("error in (no error)"=w8, "mode (read-only)"=w6, "path"=w2) -> ("error out"=→"error out":errorcluster, "ref out"=w1:T1)  [unwired: 6 in, 1 out]
  "10 Hz file ref" <- w1
  n6 = Bundle By Name(cluster="HDF5_file_refs in", "PathNow1"=w10, "PathNow2"=w3, "DateNow"=w4, "HDFRefs1.File"=w15, "HDFRefs2.File"=w13, "10HzRefs.FileRef"=w1) -> (→"HDF5_file_refs out":T2)
